vi "Create_Trajectory_Using_TrajectoryLibrary.vi"() -> ()   [LabVIEW 2019]
doc: "This utility creates trajectories based on the robot configuration, constraints and defined waypoints."
uses:
  <vilib>/Rock Robotics/WPI/ThirdParty/JAS_Junk/TrajLib/Trajectory_Library.lvlib
  <vilib>/Rock Robotics/WPI/ThirdParty/JAS_Junk/TrajLib/TypeDef/TRANSLATION2D.ctl
  <vilib>/Rock Robotics/WPI/ThirdParty/JAS_Junk/TrajLib/TypeDef/ROTATION2D.ctl
  <vilib>/Rock Robotics/WPI/ThirdParty/JAS_Junk/TrajLib/TypeDef/POSE2D.ctl
  <vilib>/Rock Robotics/WPI/ThirdParty/JAS_Junk/TrajLib/TypeDef/TRAJ_STATE.ctl
  <vilib>/Rock Robotics/WPI/ThirdParty/JAS_Junk/TrajLib/TypeDef/TRAJECTORY.ctl
  <vilib>/Rock Robotics/WPI/ThirdParty/JAS_Junk/TrajLib/TypeDef/DISPLAY_WEIGHTED_WAYPOINT.ctl
  CreateTrajectoryENUM/TrajCreateUnitsENUM.ctl
  <vilib>/Utility/miscctls.llb/LVCursorListTypeDef.ctl
  <vilib>/Rock Robotics/WPI/ThirdParty/JAS_Junk/TrajLib/TypeDef/TRAJ_CONFIG.ctl
  CreateTrajectoryTypeDef/TrajCreateConfig__V_Internal.ctl
  <vilib>/Utility/xml.llb/Read From XML File(string).vi
  <vilib>/Utility/xml.llb/Write to XML File(string).vi
  <vilib>/Utility/error.llb/DialogType.ctl
  <vilib>/Rock Robotics/WPI/ThirdParty/JAS_Junk/TrajLib/TypeDef/SIMPLE_MOTOR_FF.ctl
  <vilib>/Rock Robotics/WPI/ThirdParty/JAS_Junk/TrajLib/TypeDef/DIFF_DRIVE_KINEMATICS.ctl
panel:
  in  "Update\nConfig":bool
  out "DIFF_DRIVE_KINEMATICS":T1 {"TrackWidth_Meters" format="%20.4f"}
  in  "End Program":bool
  in  "Terminate":bool
  out "FIeldSelectorHasItems":bool
  out "IsCubic":bool
  out "outTRAJECTORY_CONFIG":T2 {"End Velocity" format="%20.4f"; "StartVelocity" format="%20.4f"; "Max Acceleration" format="%20.4f"; "MaxVelocity" format="%20.4f"}
  out "WayPoints_M":T3[](array[typedef]) {"WEIGHT" format="%13.3f"; "ANGLE" format="%13.3f"; "Y" format="%13.3f"; "X" format="%13.3f"}
  out "TRAJECTORY":T4 {"States"."POSE"."ROTATION"."SIN" format="%13.4f"; "States"."POSE"."ROTATION"."COS" format="%13.4f"; "States"."POSE"."ROTATION"."VALUE" format="%13.4f"; "States"."POSE"."TRANSLATION"."Y" format="%14.3f"; "States"."POSE"."TRANSLATION"."X" format="%14.3f"; "TotalTImeSecs" format="%20.3f"}
  in  "Tab Control":T9(tab)
  out "Read Config File Comment":string
  in  "Read Config File Name":path
  in  "ReadConfigFile":bool
  in  "Field Selector":string(combo)
  in  "Units Selector":T10
  in  "MaxVelocity":dbl=50.0 format="%17.1f"
  in  "MaxAcceleration":dbl=40.0 format="%17.1f"
  out "MaxVelocity M/S":dbl=2.0 format="%17.4f"
  out "MaxAcceleration M/S^2":dbl=1.3 format="%17.4f"
  in  "Mech Right Rear":T7={"X"=-0.5, "Y"=0.5} {"Y" format="%14.3f"; "X" format="%14.3f"}
  in  "Mech Left Rear":T7={"X"=-0.5, "Y"=-0.5} {"Y" format="%14.3f"; "X" format="%14.3f"}
  in  "Mech Right Front":T7={"X"=0.5, "Y"=0.5} {"Y" format="%14.3f"; "X" format="%14.3f"}
  in  "Mech Left Front":T7={"X"=0.5, "Y"=-0.5} {"Y" format="%14.3f"; "X" format="%14.3f"}
  in  "Use Centripetal\nAcceleration\nConstaint":bool=TRUE
  in  "Use Diff Drive\nKinematic\nConstraint":bool=TRUE
  in  "Max Voltage":dbl=12.0 format="%20.4f"
  in  "SIMPLE_MOTOR_FF":T11={"Ks"=0.9, "Kv"=0.22199, "Ka"=0.04876, "KnInv"=1.0} {"KnInv" format="%13.4f"; "Ka" format="%13.4f"; "Kv" format="%13.4f"; "Ks" format="%13.4f"}
  in  "Use Diff Drive\nVoltage\nConstraint":bool
  in  "Swerve Wheels":T7[](array[typedef])=[{"X"=0.5, "Y"=-0.5}, {"X"=0.5, "Y"=0.5}, {"X"=-0.5, "Y"=0.5}, {"X"=-0.5, "Y"=-0.5}] {"Y" format="%14.3f"; "X" format="%14.3f"}
  in  "Use Swerve Drive\nKinematics\nConstraint":bool
  in  "Use Mecanum \nDrive\nKinematics\nConstraint":bool
  out "Mech Left Front M":T7 {"Y" format="%14.3f"; "X" format="%14.3f"}
  out "Mech Right Front M":T7 {"Y" format="%14.3f"; "X" format="%14.3f"}
  out "Mech Left Rear M":T7 {"Y" format="%14.3f"; "X" format="%14.3f"}
  out "Mech Right Rear M":T7 {"Y" format="%14.3f"; "X" format="%14.3f"}
  out "SIMPLE_MOTOR_FF M":T11={"Ks"=0.0, "Kv"=0.0, "Ka"=0.0, "KnInv"=1.0} {"KnInv" format="%13.4f"; "Ka" format="%13.4f"; "Kv" format="%13.4f"; "Ks" format="%13.4f"}
  out "Swerve Wheels M":T7[](array[typedef]) {"Y" format="%14.3f"; "X" format="%14.3f"}
  in  "Track Width":dbl=20.866 format="%20.1f"
  out "Track Width M":dbl=0.66 format="%20.4f"
  in  "Max Cent Accel":dbl=20.0 format="%20.1f"
  out "Max Cent Accel M/S^2":dbl=1.0 format="%20.4f"
  in  "Use Rectangular Region\nMax Velocity Constraint":bool
  in  "Rect Reg Top Right":T7 {"Y" format="%14.3f"; "X" format="%14.3f"}
  in  "REct Reg Bot Left":T7 {"Y" format="%14.3f"; "X" format="%14.3f"}
  in  "Region Max Speed (Units/Sec)":dbl=40.0 format="%20.4f"
  out "Rect Reg Top Right M":T7 {"Y" format="%14.3f"; "X" format="%14.3f"}
  out "Rect Reg Bot Left M":T7 {"Y" format="%14.3f"; "X" format="%14.3f"}
  out "Region Max Speed M/Sec":dbl
  in  "Remove Current\nWaypoint":bool
  in  "Add New\nWaypoint":bool
  in  "WayPoints":T3[](array[typedef])=[{"X"=15.0, "Y"=105.0, "ANGLE"=-45.0, "WEIGHT"=12.0}, {"X"=105.0, "Y"=65.0, "ANGLE"=0.0, "WEIGHT"=12.0}, {"X"=210.0, "Y"=106.0, "ANGLE"=45.0, "WEIGHT"=12.0}, {"X"=350.0, "Y"=105.0, "ANGLE"=-45.0, "WEIGHT"=12.0}] {"WEIGHT" format="%13.3f"; "ANGLE" format="%13.3f"; "Y" format="%13.3f"; "X" format="%13.3f"}
  in  "Spline Type":enum32{"Radio Selection 1", "Radio Selection 2"}(radio)
  in  "Reverse":bool
  in  "UseWeights":bool
  in  "Calculate\nTrajectory":bool
  out "Trajectory\nCompleted\nError Free":bool
  out "Trajectory calculation error":errorcluster
  out "Position":cluster{dbl[], dbl[]}[](graph)
  out "Index":i32
  out "2D Picture":picture
  out "Trajectory Data":cluster{dbl[], dbl[]}[](graph)
  out "differential \ndrive \nmax speed":dbl format="%15.1f"
  out "Traj States\nSize":i32
  out "Trajectory States":T5[](array[typedef]) {"POSE"."ROTATION"."SIN" format="%13.4f"; "POSE"."ROTATION"."COS" format="%13.4f"; "POSE"."ROTATION"."VALUE" format="%13.4f"; "POSE"."TRANSLATION"."Y" format="%14.3f"; "POSE"."TRANSLATION"."X" format="%14.3f"}
  in  "Trajectory JSON File Name":path
  in  "PathWeaver Length Units":T12(radio)
  in  "WriteJSONFile":bool
  in  "Trajectory Type":enum32{"Radio Selection 1", "Radio Selection 2"}(radio)
  in  "Trajectory File Comment":string
  in  "Trajectory CSV File Name":path
  in  "WriteTrajFile":bool
  in  "Write Config File Comment":string
  in  "Write Config File Name":path
  in  "WriteConfigFile":bool
  # "Create Trajectory  (Use LabVIEW trajectory library)"
  # "Instructions:  \n----------------\n\nThis utility will create a trajectory, show the data on the various tabs, and optionally write a \"field absolute\" or \"robot relative\" trajectory to a file. \nTo use this utility:\n\n    1) Read all of these instructions!\n    2) Define the robot's physical data on the \"Robot Data\" tab.  \n    3) Define the robot's movement constraints on the \"Constraints\" and \"Constraints 2\" tab.  \n    4) Define the trajectory on the \"Define/Create Trajectory\" tab.  These are the beginning and ending positions/headings, and internal positions/headings.  \n         Cubic splines only use the first and last \"angle\".  The other internal \"angles\" are calculated.  Quintic splines use all the defined angles.\n    5) Press the \"Calculate Trajectory\".  If a good trajectory was calculated it will be displayed.  If no errors are generated the Trajectory Complete\n         light will be on.  Errors will be displayed in the error indicator.  The path can be recalculated many times before performing any other action.\n\nAfter a Trajectory has been calculated, the \"trajectory can be written to a file.  The absolute path is converted to a robot relative trajectory.  To do this:\n    1) Enter a comment to be included in the file.  Anything can be entered.\n    2) Select the file name.\n    3) Press \"Create CSV Trajectory File\"  If an error occurs it will be displayed in the File Creation Error indicator.\n\nTo:\n  --  Move a WayPoint  -- Left click the waypoint and drag it using the mouse.\n  --  Rotate a WayPoint  -- Left click the waypoint to select, then use the mouse wheel to increase or decrease the heading\n  --  Change WayPoint weight  -- Left click the waypoint to select, then use CTRL key and mouse wheel to increase or decrease the weight.\n\nNotes:\n--------\n- All the robot parameters, path, and field dimensions are in UNITS, and DEGREES.  Select UNITS from the \"Robot Data\" page.  The resulting  \n  trajectory is converted to METERS, and RADIANS to match the rest of this library!\n- 2019 playing field size - width: 26 ft 11.25 In = 323.25 in , length: 52 ft 5.25 in = 629.25 in  (This changes from year to year.  Larger fields are allowed.)\n\nAcknowlegements\n------------------------\n- Nathanael Cornell from FRC team 5205 added the initial code to visually move and rotate waypoints."
  # "Read Trajectory Waypoints and Configuration from File"
  # "ROBOT DATA"
  # "UNITS/SEC"
  # "Meters/SEC"
  # "UNITS/SEC^2"
  # "Meters/SEC^2"
  # "Simulated diff drive robot max speed is: 68.266 Inches/Second"
  # "UTILITY CONFIGURATION"
  # "Diff Kinematics Constraint"
  # "Centripetal Accel Constraint"
  # "Diff Voltage Constraint"
  # "UNITS"
  # "UNITS/SEC^2"
  # "VOLTS"
  # "METERS"
  # "METERS/SEC^2"
  # "Distance is:\nUNITS"
  # "Simulated robot wheelbase is 20.87 in"
  # "Ks = Volts\nKv = VoltSec/Meter\nKa = Volt(Sec^2)/Meter"
  # "Swerve Kinematics Constraint"
  # "Mechanum Kinematics Constraint"
  # "Values\nare \nUNITS"
  # "Values\nare \nUNITS"
  # "Rectangular Region Constraint  - Max Velocity Constraint"
  # "Values\nare \nUNITS"
  # "TRAJECTORY DEFINITION"
  # "To delete array elements or the entire array, right click on the array or element, select Data Operations, then select the action to be performed."
  # "UNITS, UNITS, DEGREES, SCALAR"
  # "INCHES/SEC"
  # "Write Trajectory to File   -   CSV, and / or JSON"
  # "Write Trajectory Waypoints and Configuration to File"
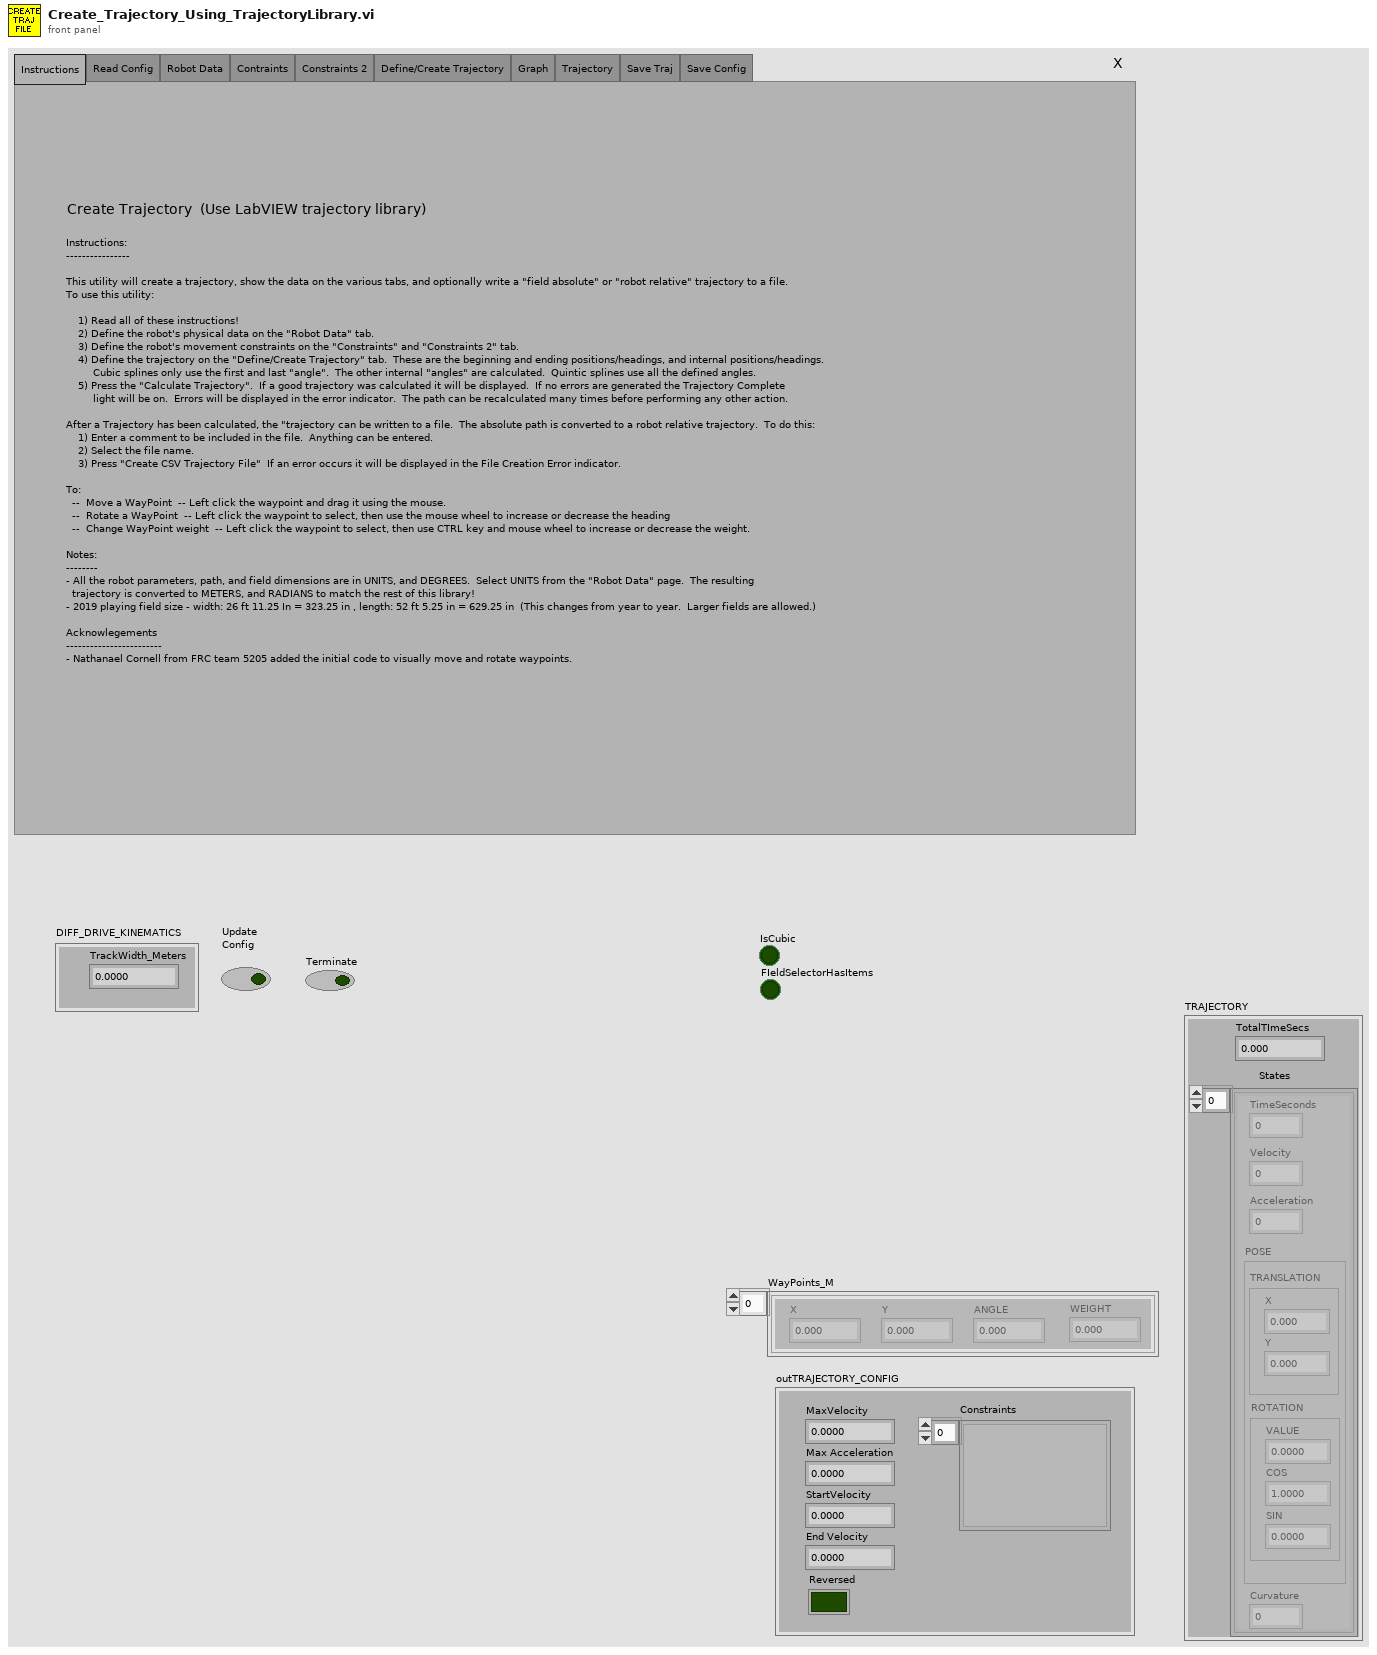
[diagram p1: front panel]
types:
  T1 = typedef "Trajectory_Library.lvlib/DIFF_DRIVE_KINEMATICS.ctl" = cluster{"TrackWidth_Meters":dbl}
  T2 = typedef "Trajectory_Library.lvlib/TRAJ_CONFIG.ctl" = cluster{"MaxVelocity":dbl, "Max Acceleration":dbl, "StartVelocity":dbl, "End Velocity":dbl, "Reversed":bool, "Constraints":variant[]}
  T3 = typedef "Trajectory_Library.lvlib/DISPLAY_WEIGHTED_WAYPOINT.ctl" = cluster{"X":dbl, "Y":dbl, "ANGLE":dbl, "WEIGHT":dbl}
  T4 = typedef "Trajectory_Library.lvlib/TRAJECTORY.ctl" = cluster{"TotalTImeSecs":dbl, "States":T5[]}
  T5 = typedef "Trajectory_Library.lvlib/TRAJ_STATE.ctl" = cluster{"TimeSeconds":dbl, "Velocity":dbl, "Acceleration":dbl, "POSE":T6, "Curvature":dbl}
  T6 = typedef "Trajectory_Library.lvlib/POSE2D.ctl" = cluster{"TRANSLATION":T7, "ROTATION":T8}
  T7 = typedef "Trajectory_Library.lvlib/TRANSLATION2D.ctl" = cluster{"X":dbl, "Y":dbl}
  T8 = typedef "Trajectory_Library.lvlib/ROTATION2D.ctl" = cluster{"VALUE":dbl, "COS":dbl, "SIN":dbl}
  T9 = enum32{"Instructions", "Read Config", "Robot Data", "Contraints", "Constraints 2", "Define/Create Trajectory", "Graph", "Trajectory", "Save Traj", "Save Config"}
  T10 = typedef "TrajCreateUnitsENUM.ctl" = enum16{"Inches", "Feet", "Centimeters", "Meters"}
  T11 = typedef "Trajectory_Library.lvlib/SIMPLE_MOTOR_FF.ctl" = cluster{"Ks":dbl, "Kv":dbl, "Ka":dbl, "KnInv":dbl}
  T12 = enum32{"Radio Selection 1", "Radio Selection 2", "Radio Selection 3", "Radio Selection 4", "Radio Selection 5"}
  T13 = typedef "LVCursorListTypeDef.ctl" = cluster{"Name":string, "Color":u32, "Style":u8, "Point Style":u8, "Name Visible":bool, "Allow Drag":bool, "Cursor Mode":u32, "Plot":i32, "Index":i32, "Position":cluster{"X":dbl, "Y":dbl}, "X Scale":u32, "Y Scale":u32, "Watch Plots":i32[], "Watch All Plots":bool, "Plot Area":i32, "Label Offset":cluster{"X":dbl, "Y":dbl}}[]
  T14 = enum8{"Enabled", "Disabled", "Disabled and Grayed Out"}
  T15 = cluster{"Name":string, "Color":u32, "Style":u8, "Point Style":u8, "Name Visible":bool, "Allow Drag":bool, "Cursor Mode":u32, "Plot":i32, "Index":i32, "Position":cluster{"X":dbl, "Y":dbl}, "X Scale":u32, "Y Scale":u32, "Watch Plots":i32[], "Watch All Plots":bool, "Plot Area":i32, "Label Offset":cluster{"X":dbl, "Y":dbl}}
  T16 = typedef "TrajCreateConfig__V_Internal.ctl" = cluster{"Write Config File Name":path, "Write Config File Comment":string, "WayPoints":T3[], "TRAJECTORY_CONFIG":T2, "IsCubic":bool, "Units Selector":T10, "UseWeights":bool, "FieldName":string}
  T17 = typedef "Trajectory_Library.lvlib/SWERVE_DRIVE_KINEMATICS.ctl" = cluster{"NumModules":i32, "InverseKinematics":T18, "ForwardKinematics":T18, "Modules":T7[], "PrevCoR":T7, "SavedModuleStates":T19[]}
  T18 = typedef "NI_Matrix.lvlib/RealMatrix.ctl" = dbl[][]
  T19 = typedef "Trajectory_Library.lvlib/SWERVE_DRIVE_MODULE_STATE.ctl" = cluster{"Speed":dbl, "Angle":T8}
  T20 = typedef "Trajectory_Library.lvlib/MECA_DRIVE_KINEMATICS.ctl" = cluster{"FrontLeft":T7, "FrontRight":T7, "RearLeft":T7, "RearRight":T7, "InverseKinematics":T18, "ForwardKinematics":T18, "PrevCoR":T7}
  T21 = typedef "Trajectory_Library.lvlib/TRAJ_CONSTRAINT_MAX_VELOCITY.ctl" = cluster{"Max Velocity":dbl, "IM UNIQUE":bool}
  T22 = typedef "Trajectory_Library.lvlib/TRAJ_CONSTRAINT_RECT_REGION.ctl" = cluster{"BottomLeftPoint":T7, "TopRightPoint":T7, "Constraint":variant, "Constraint Type":T23}
  T23 = typedef "Trajectory_Library.lvlib/TRAJ_CONSTRAINT_TYPES_ENUM.ctl" = enum16{"UNDEFINED", "DIFF DRIVE KINEMATICS", "DIFF DRIVE VOLTAGE", "CENTRIPITAL ACCEL", "MECA DRIVE KINEMATICS", "SWERVE DRIVE KINEMATICS", "MAXIMUM VELOCITY", "ELLIPTICAL REGION", "RECTANGULAR REGION"}
  T24 = typedef "DialogType.ctl" = u16
  T25 = typedef "Trajectory_Library.lvlib/TRAJ_CONSTRAINT_DIIF_DRIVE_KINEMATICS.ctl" = cluster{"Max Speed (M/S)":dbl, "DIFF_DRIVE_KINEMATICS":T1, "Max Accel (M/S2)":dbl}
  T26 = typedef "Trajectory_Library.lvlib/TRAJ_CONSTRAINT_CENTRIPETAL_ACCEL.ctl" = cluster{"Max Cent Accel":dbl}
  T27 = typedef "Trajectory_Library.lvlib/TRAJ_CONSTRAINT_DIIF_DRIVE_VOLTAGE.ctl" = cluster{"Max Voltage":dbl, "DIFF_DRIVE_KINEMATICS":T1, "SIMPLE_MOTOR_FF":T11}
  T28 = typedef "Trajectory_Library.lvlib/TRAJ_CONSTRAINT_MECA_DRIVE_KINEMATICS.ctl" = cluster{"Max Speed (M/S)":dbl, "MECA_DRIVE_KINEMATICS":T20}
  T29 = typedef "Trajectory_Library.lvlib/TRAJ_CONSTRAINT_SWERVE_DRIVE_KINEMATICS.ctl" = cluster{"Max Speed (M/S)":dbl, "SwerveKinematics":T17}
  T30 = typedef "TrajCreateConfig_V5.ctl" = cluster{"Write Config File Name":path, "Write Config File Comment":string, "WayPoints":T3[], "TRAJECTORY_CONFIG_V4":T31, "IsCubic":bool, "Units Selector":T10, "UseWeights":bool, "FieldName":string, "Rect Region Exists":bool, "RectRegionBotLeft":T7, "RectRegionTopRight":T7, "Rect Region Max Speed":dbl}
  T31 = typedef "TrajCreateTrajConfig_V4.ctl" = cluster{"MaxVelocity":dbl, "Max Acceleration":dbl, "StartVelocity":dbl, "End Velocity":dbl, "Reversed":bool, "DiffDrKineConstntDefined":bool, "CentAcellConstntDefined":bool, "DiffDrVoltConstntDefined":bool, "DIFF_DRIVE_KINE_CONSTRAINT":T25, "CENTRIPETAL_ACCEL_CONSTRAINT":T26, "SwerveDrKineConstntDefined":bool, "SWERVE_DRIVE_KINE_CONSTRAINT":T29, "DIFF_DRIVE_VOLTAGE_CONSTRAINT":T27, "MECANUM_DRIVE_KINE_CONSTRAINT":T28, "MecanumDrKineConstntDefined":bool}
  T32 = cluster{"Shift":bool, "Ctrl":bool, "Alt":bool, "Cmd":bool, "Opt":bool}
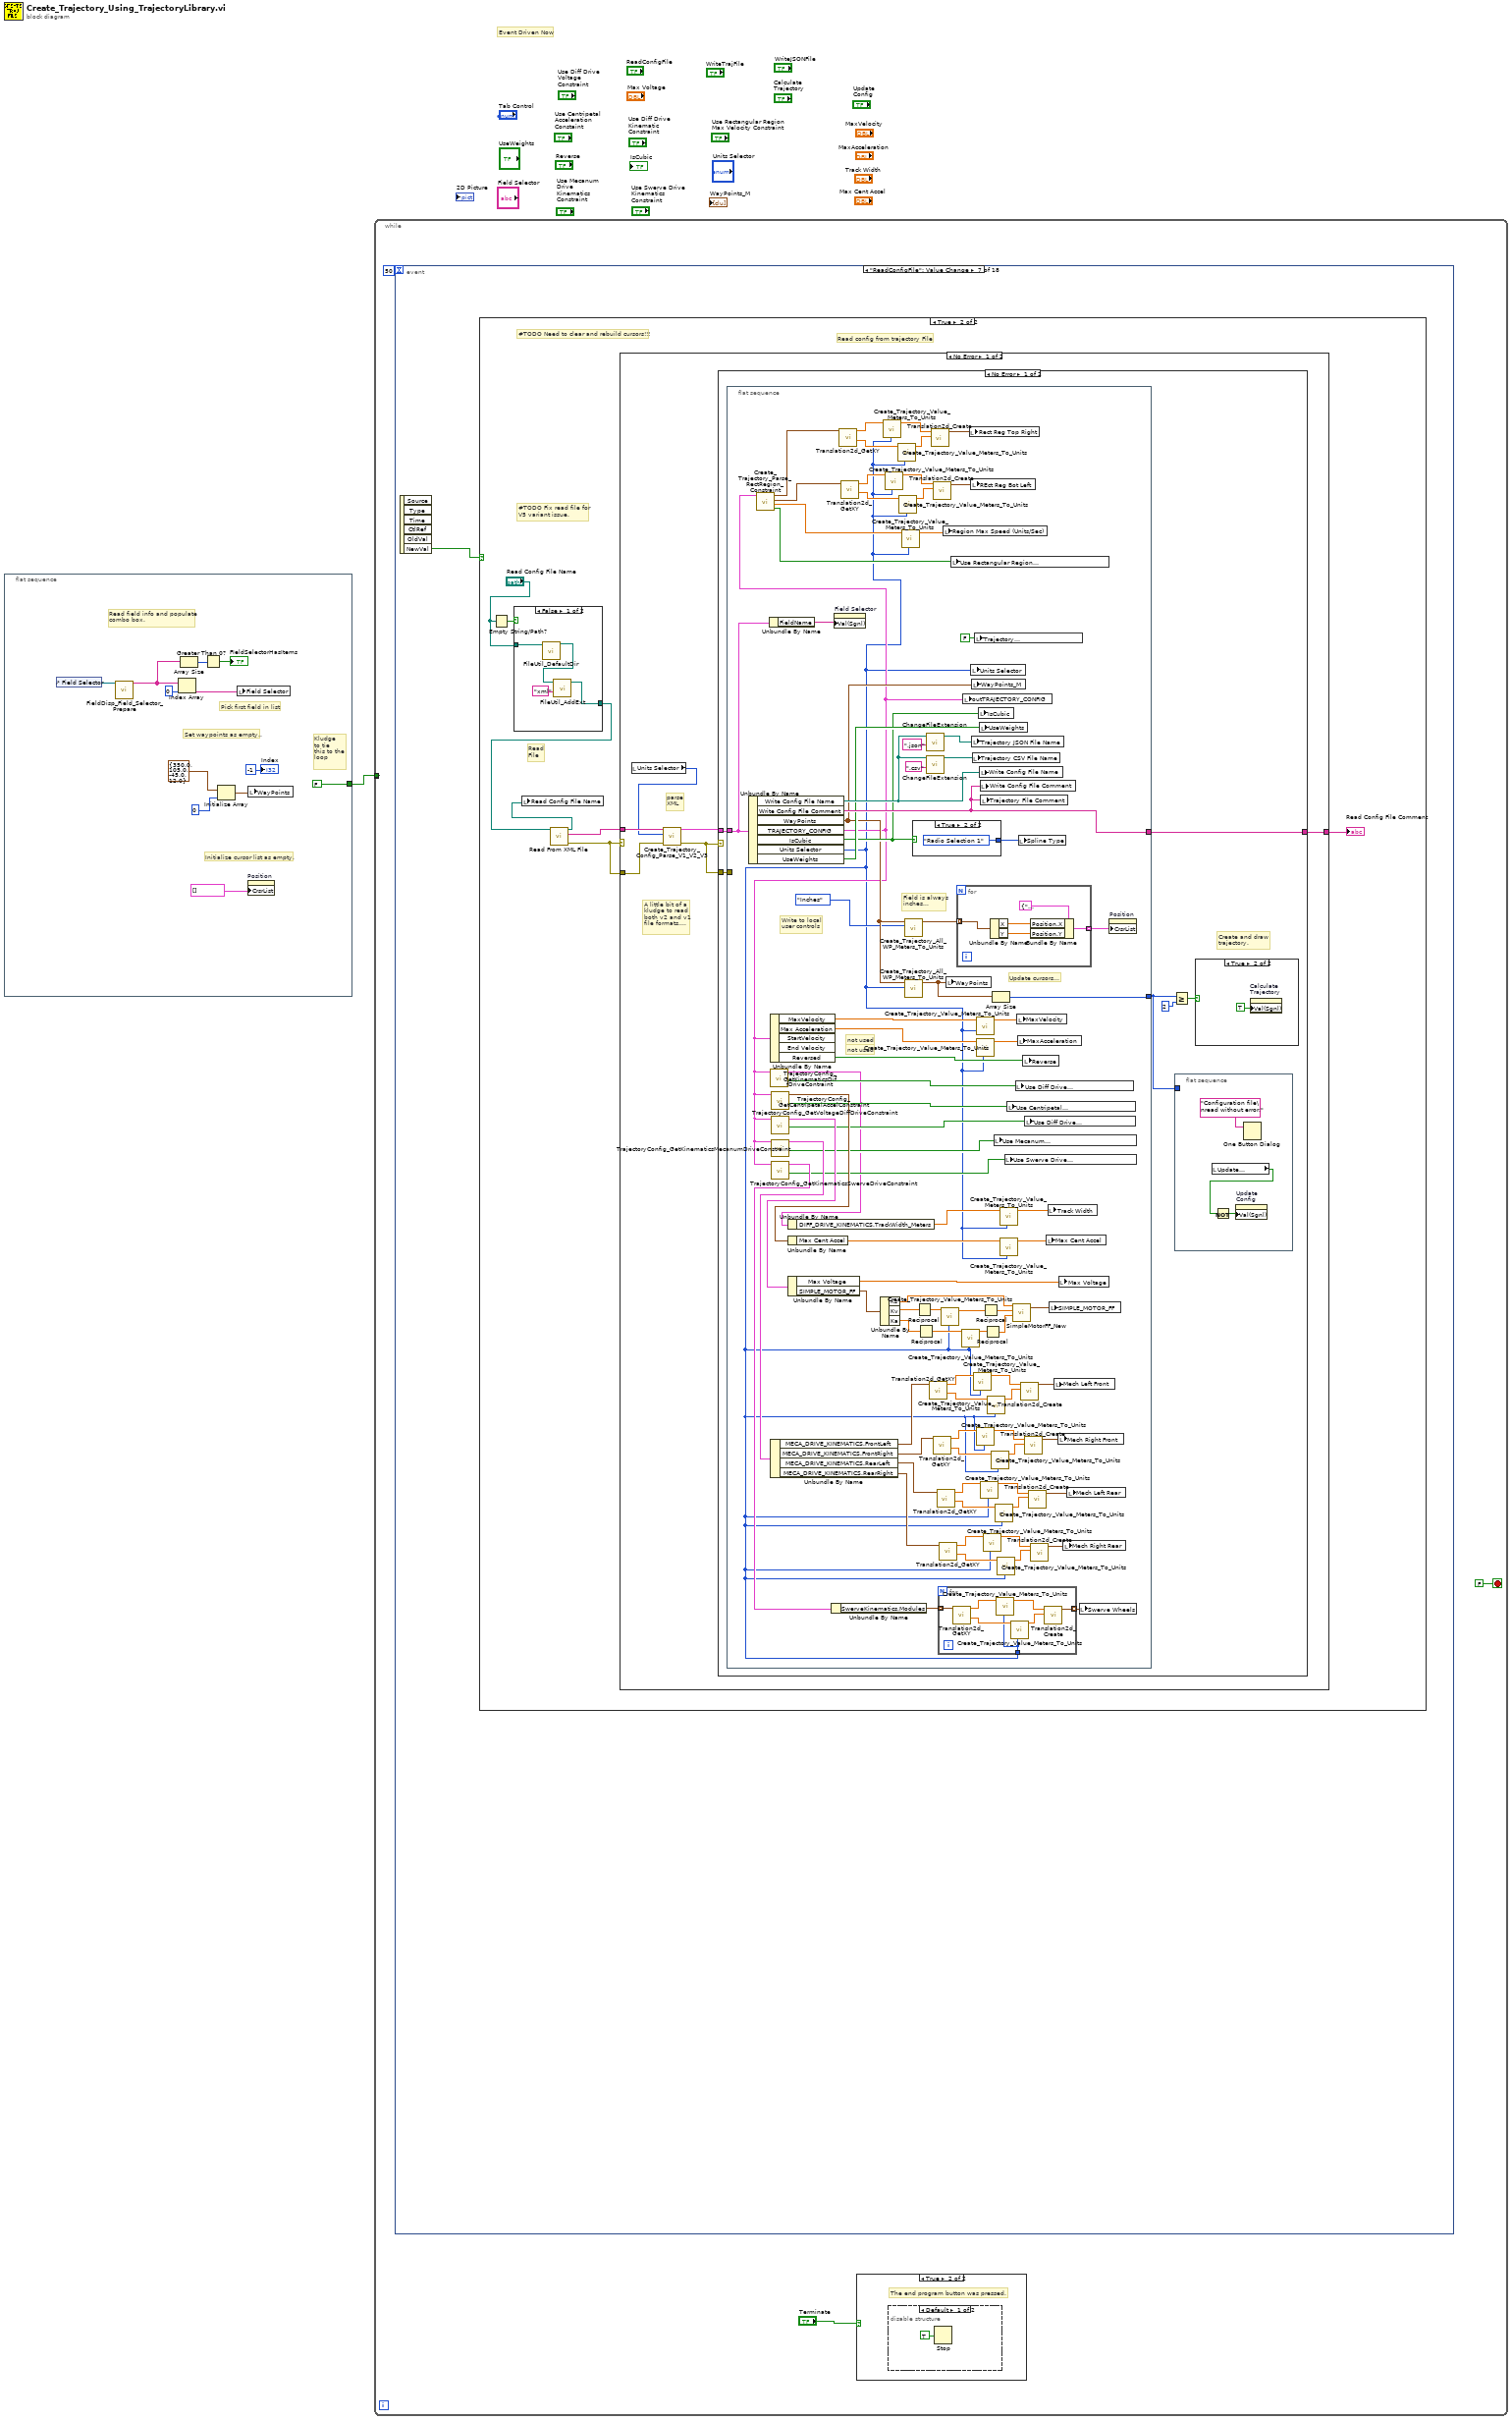
[diagram p0: block diagram]
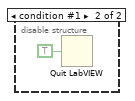
[diagram p3: hidden frame]
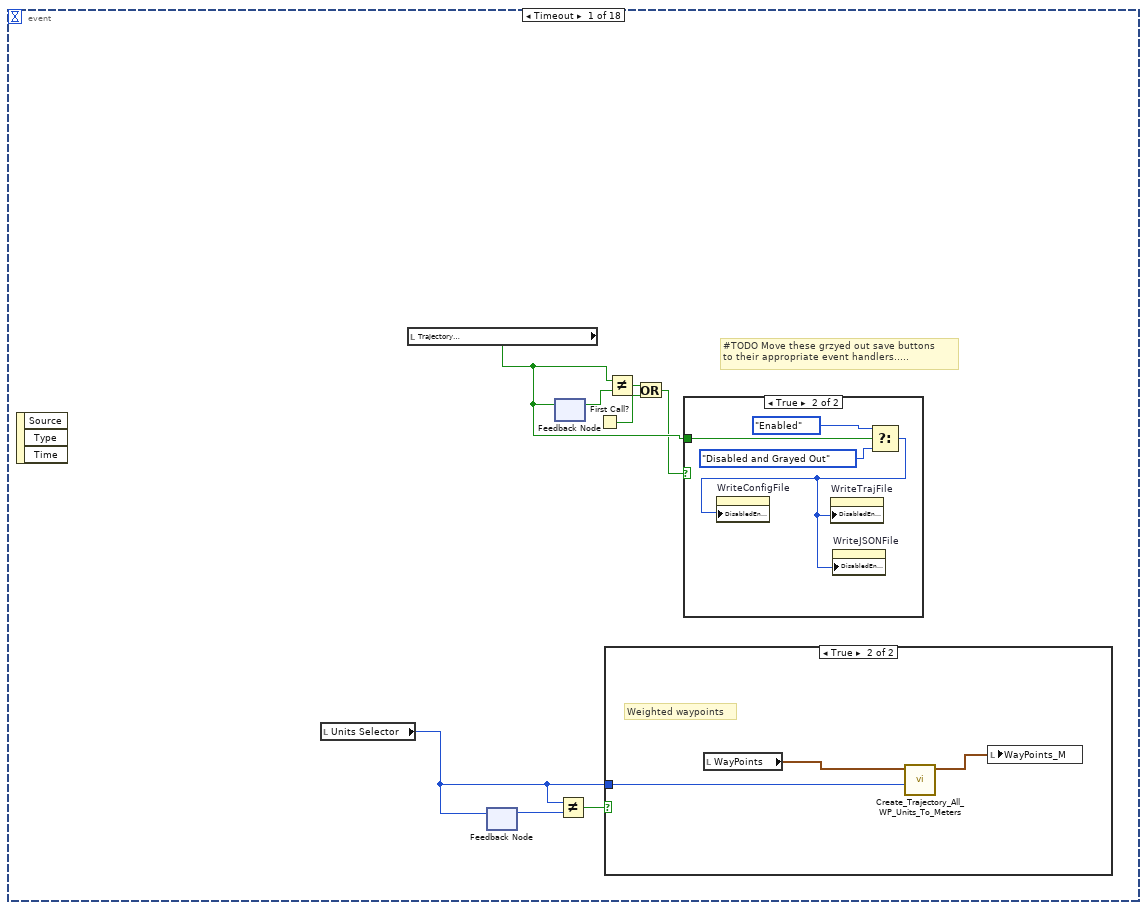
[diagram p4: hidden frame]
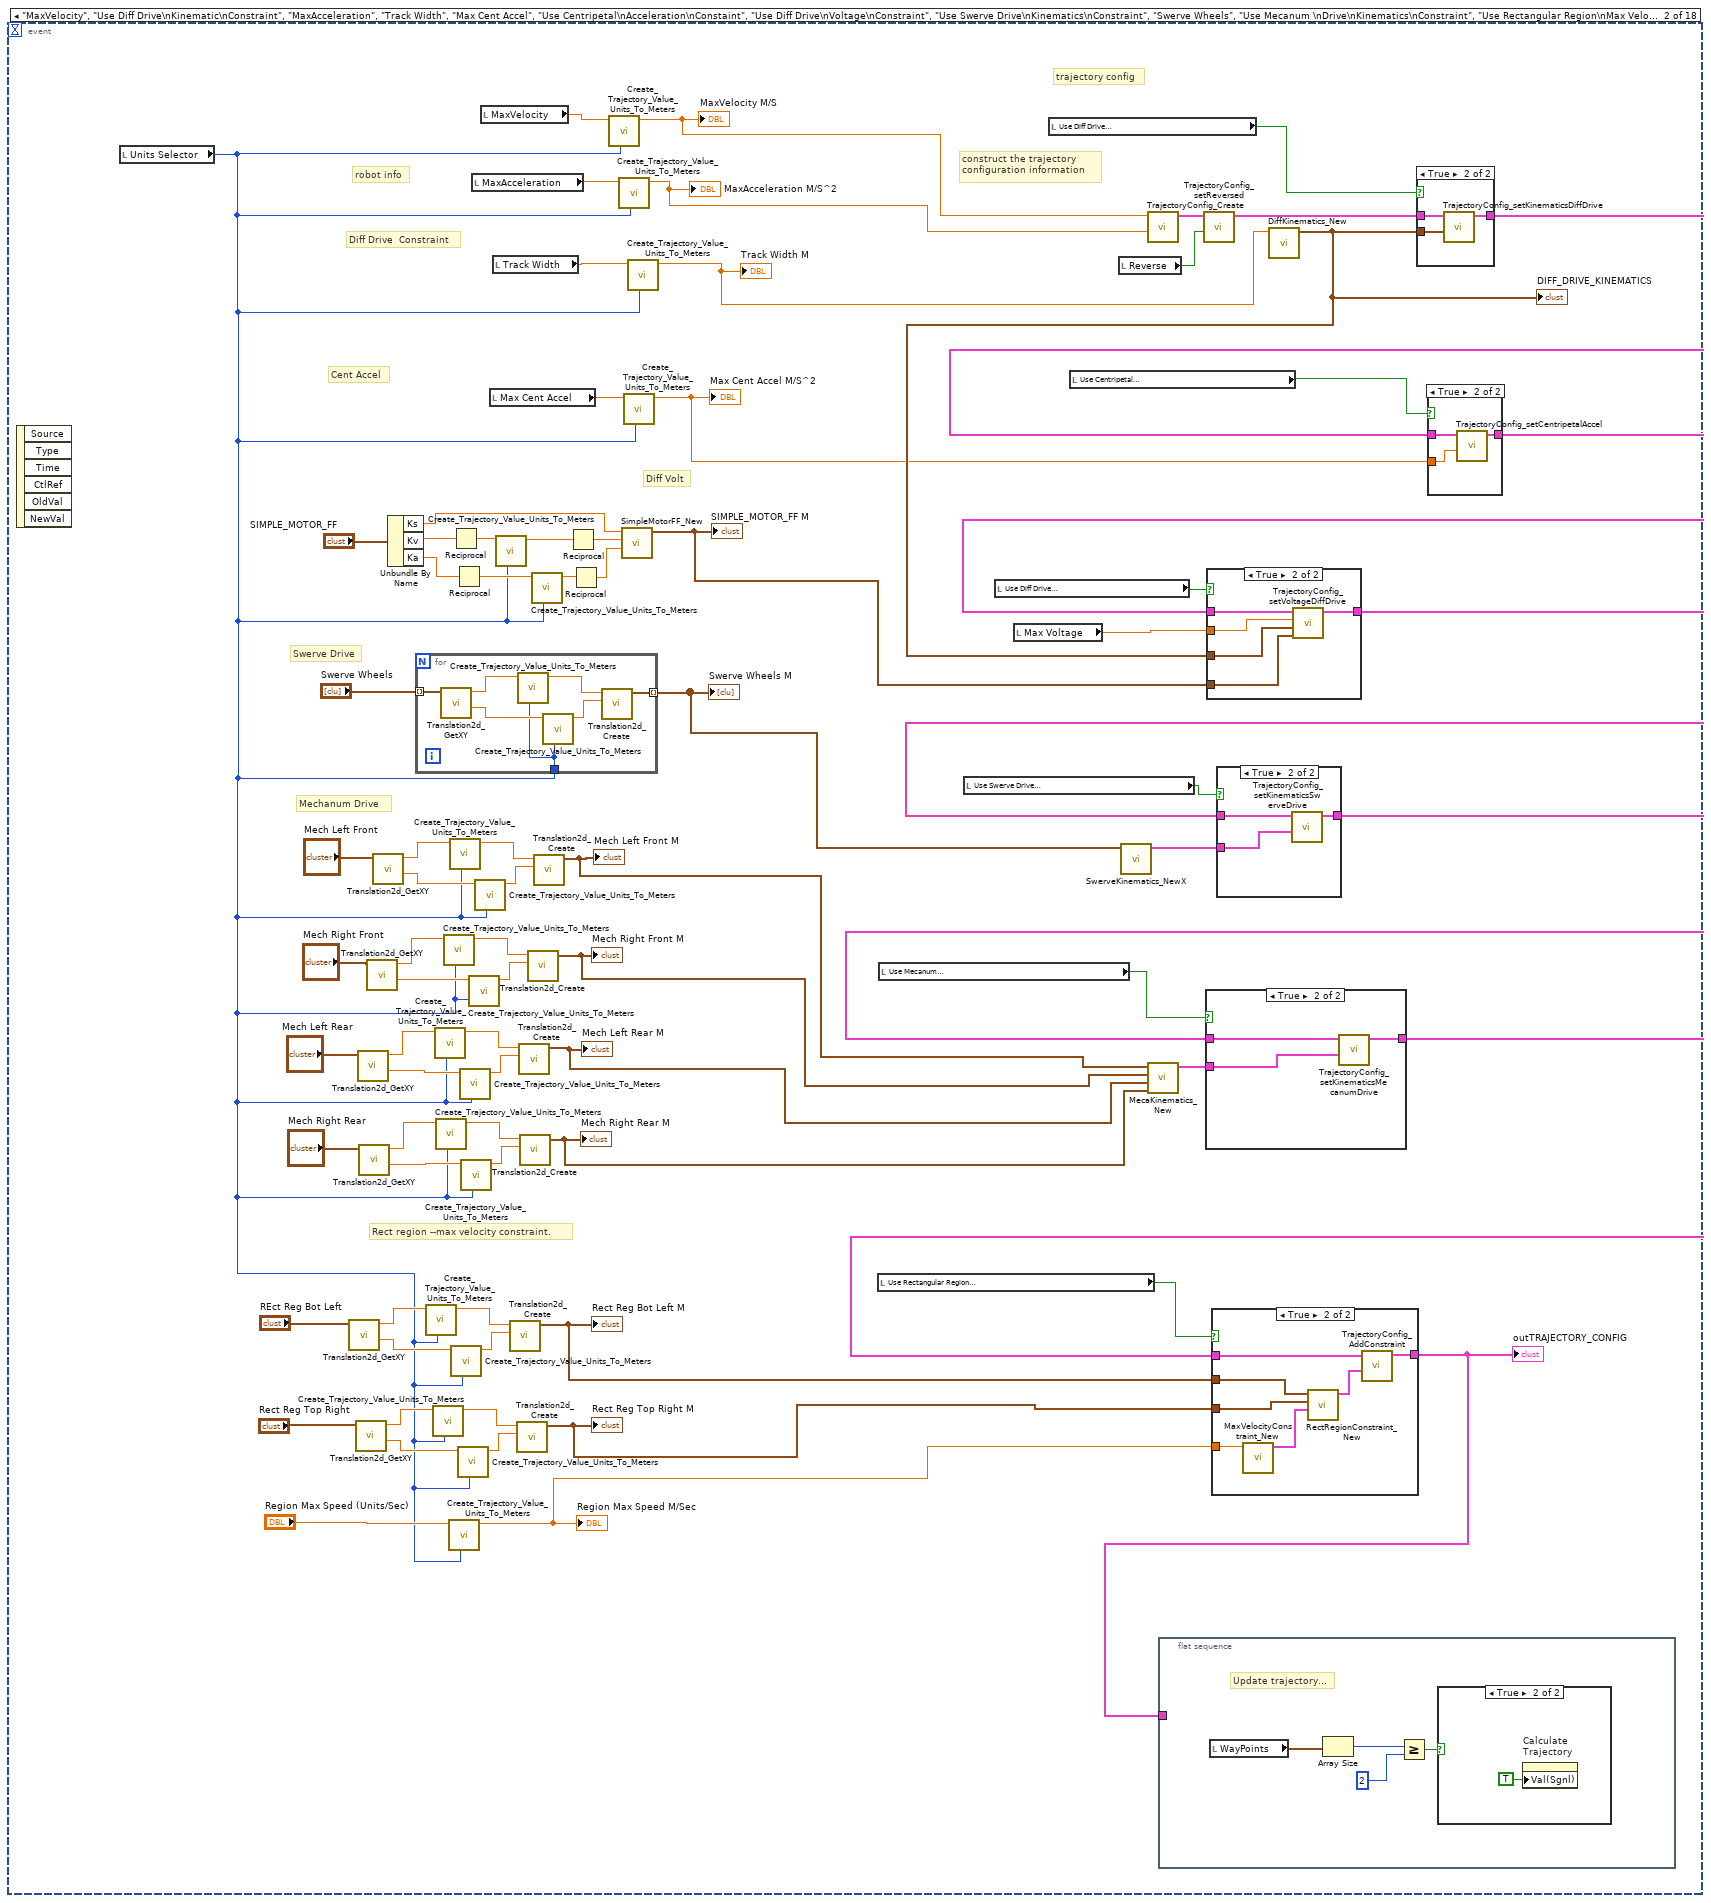
[diagram p7: hidden frame]
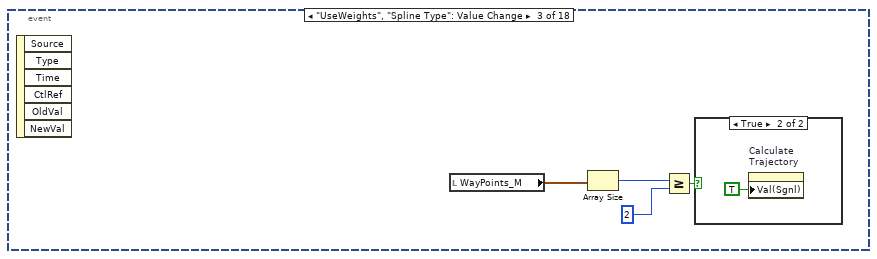
[diagram p15: hidden frame]
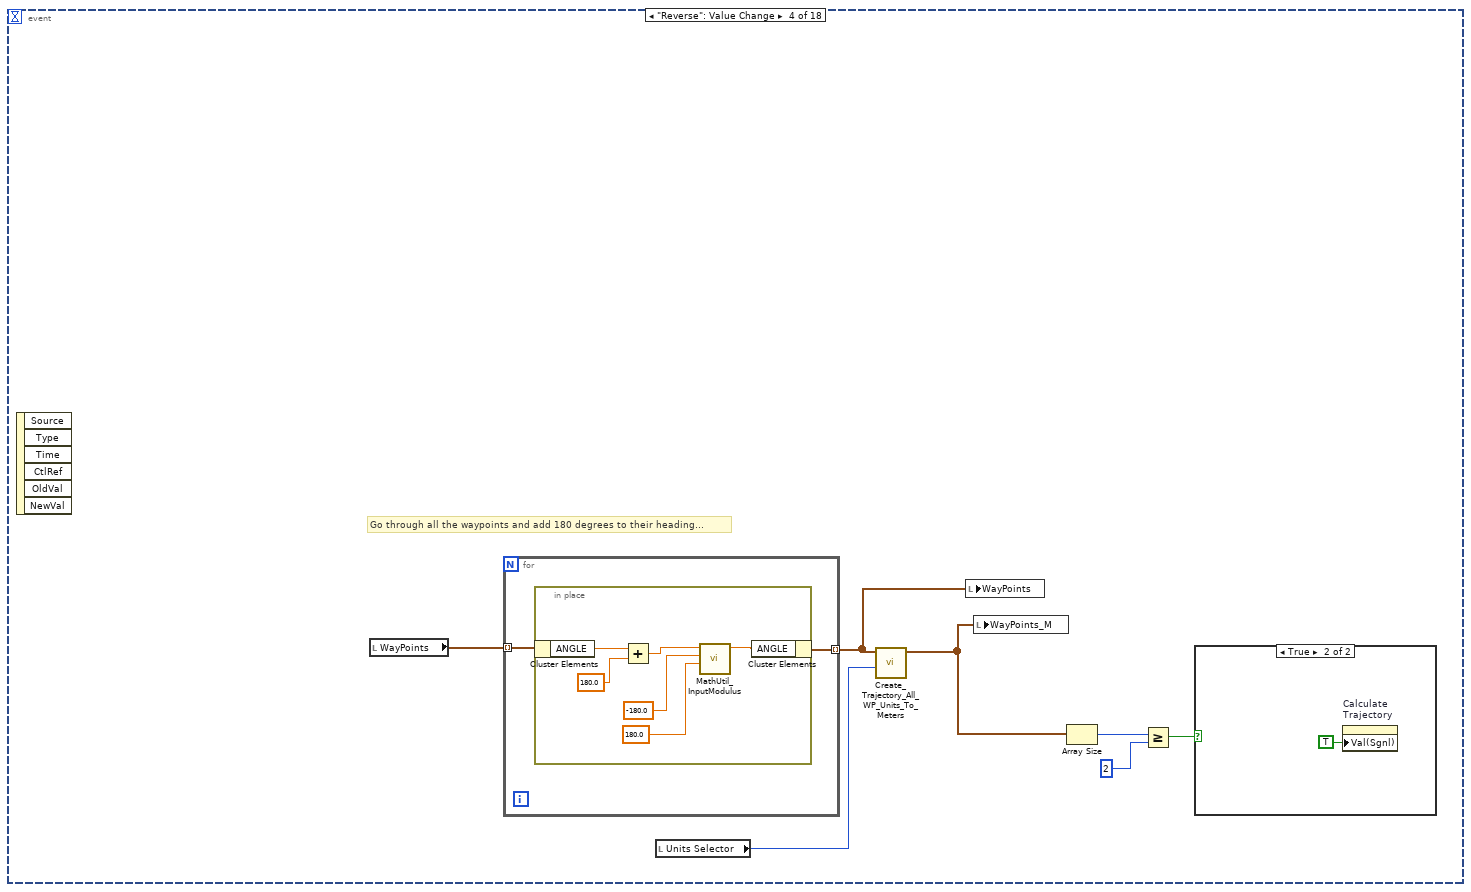
[diagram p17: hidden frame]
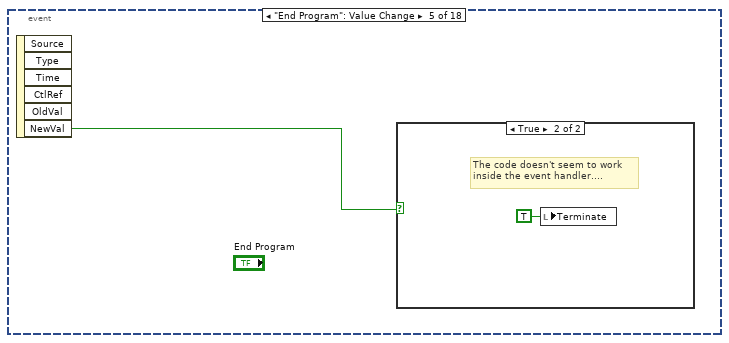
[diagram p19: hidden frame]
diagram:
  # "Event Driven Now"
  n1 = flat-sequence {
    tunnel: [FALSE] -> w1
    frame #0 {
      # "Pick first field in list"
      # "Read field info and populate\ncombo box."
      # "Kludge\nto tie\nthis to the\nloop"
      # "Initialize cursor list as empty."
      # "Set waypoints as empty.."
      n2 = control-ref of="Field Selector"() -> (w6:refnum<vi>)
      n3 = call <vilib>:"FieldDisp_Field_Selector_Prepare.vi"("ComboBox Ref"=w6) -> ("section names"=w7:string[])  [unwired: 9 in, 1 out]
      n4 = Index Array(array=w7, index=0) -> (element=w5:string)
      n5 = Array Size(array=w7) -> (size(s)=w3:i32)
      n6 = Greater Than 0?(x=w3) -> (x > 0?=→"FIeldSelectorHasItems":bool)
      n7 = Initialize Array(T3 {"X"=350.0, "Y"=105.0, "ANGLE"=-45.0, "WEIGHT"=12.0} ("path"), 0 ("dimension size")) -> (w11:T3[])
      n8 = local write "Field Selector"(w5) -> ()
      n9 = property on="Position" class="XYGraph (strict)"("CrsrList"=T13 [] ("Cursor List")) -> ()  [unwired: 2 in, 2 out]
      n10 = local write "WayPoints"(w11) -> ()
      "Index" <- -1 ("Index")
    }
  }
  n11 = while {
    tunnel: [w15] -> _
    tunnel: w1 -> [w15]
    stop <- FALSE stop-if-true
    n12 = event shown="[6] \"ReadConfigFile\": Value Change" {
      selector: _ -> [_ _ _ _ _ _ _ _ _ _ _ _ _ _ _ _ _ _]
      dyn-events: _ -> [_ _ _ _ _ _ _ _ _ _ _ _ _ _ _ _ _ _]
      timeout: 50 -> [_ _ _ _ _ _ _ _ _ _ _ _ _ _ _ _ _ _]
      event Timeout {
        # "#TODO Move these grzyed out save buttons\nto their appropriate event handlers....."
        n13 = event-data() -> ()  [unwired: 1 in, 3 out]
        n14 = local read "Units Selector"() -> (w20:T10)
        n15 = local read "Trajectory\nCompleted\nError Free"() -> (w27:bool)
        n16 = feedback-in #1(w20) -> ()
        n17 = feedback #1() -> (w21:T10)  [unwired: 1 in]
        n18 = feedback #2() -> (w23:bool)  [unwired: 1 in]
        n19 = feedback-in #2(w27) -> ()
        n20 = Not Equal?(x=w20, y=w21) -> (x != y?=w22:bool)
        n21 = First Call?() -> (First Call?: T/F=w25:bool)
        n22 = case shown="True" w22 {
          tunnel: w20 -> [_ w30]
          frame False {
          }
          frame True {
            # "Weighted waypoints"
            n23 = local read "WayPoints"() -> (w28:T3[])
            n24 = call "Create_Trajectory_All_WP_Units_To_Meters.vi"("Units Selector"=w30, "WayPoints"=w28) -> ("Array"=w29:T3[])  [unwired: 9 in]
            n25 = local write "WayPoints_M"(w29) -> ()
          }
        }
        n26 = Not Equal?(x=w27, y=w23) -> (x != y?=w24:bool)
        n27 = Or(x=w24, y=w25) -> (x .or. y?=w26:bool)
        n28 = case shown="True" w26 {
          tunnel: w27 -> [_ w34]
          frame False {
          }
          frame True {
            n29 = Select(t=T14."Enabled" ("Disabled"), s=w34, f=T14."Disabled and Grayed Out" ("Disabled")) -> (s? t:f=w31:T14)
            n30 = property on="WriteConfigFile" class="Bool"("DisabledEnum"=w31) -> ()  [unwired: 2 in, 2 out]
            n31 = property on="WriteTrajFile" class="Bool (strict)"("DisabledEnum"=w31) -> ()  [unwired: 2 in, 2 out]
            n32 = property on="WriteJSONFile" class="Bool (strict)"("DisabledEnum"=w31) -> ()  [unwired: 2 in, 2 out]
          }
        }
      }
      event "MaxVelocity", "Use Diff Drive\nKinematic\nConstraint", "MaxAcceleration", "Track Width", "Max Cent Accel", "Use Centripetal\nAcceleration\nConstaint", "Use Diff Drive\nVoltage\nConstraint", "Use Swerve Drive\nKinematics\nConstraint", "Swerve Wheels", "Use Mecanum \nDrive\nKinematics\nConstraint", "Use Rectangular Region\nMax Velocity Constraint", "Region Max Speed (Units/Sec)", "Max Voltage", "Update\nConfig": Value Change {
        # "construct the trajectory\nconfiguration information"
        # "Rect region --max velocity constraint."
        # "Swerve Drive"
        # "Mechanum Drive"
        # "Diff Volt"
        # "Cent Accel"
        # "robot info"
        # "Diff Drive  Constraint"
        # "trajectory config"
        n33 = event-data() -> ()  [unwired: 1 in, 6 out]
        n34 = local read "Units Selector"() -> (w67:T10)
        n35 = call <vilib>:"Translation2d_GetXY.vi"("In Translation"="REct Reg Bot Left") -> ("Y"=w77:dbl, "X"=w75:dbl)  [unwired: 9 in]
        n36 = call <vilib>:"Translation2d_GetXY.vi"("In Translation"="Rect Reg Top Right") -> ("Y"=w73:dbl, "X"=w71:dbl)  [unwired: 9 in]
        n37 = call <vilib>:"Translation2d_GetXY.vi"("In Translation"="Mech Left Rear") -> ("Y"=w91:dbl, "X"=w89:dbl)  [unwired: 9 in]
        n38 = call <vilib>:"Translation2d_GetXY.vi"("In Translation"="Mech Right Rear") -> ("Y"=w96:dbl, "X"=w94:dbl)  [unwired: 9 in]
        n39 = call <vilib>:"Translation2d_GetXY.vi"("In Translation"="Mech Right Front") -> ("Y"=w86:dbl, "X"=w84:dbl)  [unwired: 9 in]
        n40 = call <vilib>:"Translation2d_GetXY.vi"("In Translation"="Mech Left Front") -> ("Y"=w81:dbl, "X"=w79:dbl)  [unwired: 9 in]
        n41 = Unbundle By Name("SIMPLE_MOTOR_FF") -> ("Ks"=w101:dbl, "Kv"=w102:dbl, "Ka"=w109:dbl)
        n42 = for {
          tunnel: "Swerve Wheels" -> [w151] mode=indexing
          tunnel: [w150] -> w48 mode=indexing
          tunnel: w67 -> [w149]
          n43 = call <vilib>:"Translation2d_GetXY.vi"("In Translation"=w151) -> ("Y"=w153:dbl, "X"=w155:dbl)  [unwired: 9 in]
          n44 = call "Create_Trajectory_Value_Units_To_Meters.vi"("Units Selector"=w149, "Units"=w155) -> ("Meters"=w154:dbl)  [unwired: 9 in]
          n45 = call "Create_Trajectory_Value_Units_To_Meters.vi"("Units Selector"=w149, "Units"=w153) -> ("Meters"=w152:dbl)  [unwired: 9 in]
          n46 = call <vilib>:"Translation2d_Create.vi"("Y"=w152, "X"=w154) -> ("TRANSLATION"=w150:T7)  [unwired: 9 in]
        }
        "Swerve Wheels M" <- w48
        n47 = call "Create_Trajectory_Value_Units_To_Meters.vi"("Units Selector"=w67, "Units"=w75) -> ("Meters"=w76:dbl)  [unwired: 9 in]
        n48 = call "Create_Trajectory_Value_Units_To_Meters.vi"("Units Selector"=w67, "Units"=w71) -> ("Meters"=w72:dbl)  [unwired: 9 in]
        n49 = call "Create_Trajectory_Value_Units_To_Meters.vi"("Units Selector"=w67, "Units"=w89) -> ("Meters"=w90:dbl)  [unwired: 9 in]
        n50 = call "Create_Trajectory_Value_Units_To_Meters.vi"("Units Selector"=w67, "Units"=w94) -> ("Meters"=w95:dbl)  [unwired: 9 in]
        n51 = call "Create_Trajectory_Value_Units_To_Meters.vi"("Units Selector"=w67, "Units"=w84) -> ("Meters"=w85:dbl)  [unwired: 9 in]
        n52 = call "Create_Trajectory_Value_Units_To_Meters.vi"("Units Selector"=w67, "Units"="Region Max Speed (Units/Sec)") -> ("Meters"=w36:dbl)  [unwired: 9 in]
        "Region Max Speed M/Sec" <- w36
        n53 = call "Create_Trajectory_Value_Units_To_Meters.vi"("Units Selector"=w67, "Units"=w79) -> ("Meters"=w80:dbl)  [unwired: 9 in]
        n54 = Reciprocal(x=w102) -> (1/x=w103:dbl)
        n55 = call "Create_Trajectory_Value_Units_To_Meters.vi"("Units Selector"=w67, "Units"=w77) -> ("Meters"=w78:dbl)  [unwired: 9 in]
        n56 = Reciprocal(x=w109) -> (1/x=w106:dbl)
        n57 = call "Create_Trajectory_Value_Units_To_Meters.vi"("Units Selector"=w67, "Units"=w73) -> ("Meters"=w74:dbl)  [unwired: 9 in]
        n58 = call "Create_Trajectory_Value_Units_To_Meters.vi"("Units Selector"=w67, "Units"=w91) -> ("Meters"=w92:dbl)  [unwired: 9 in]
        n59 = call "Create_Trajectory_Value_Units_To_Meters.vi"("Units Selector"=w67, "Units"=w96) -> ("Meters"=w97:dbl)  [unwired: 9 in]
        n60 = call "Create_Trajectory_Value_Units_To_Meters.vi"("Units Selector"=w67, "Units"=w86) -> ("Meters"=w87:dbl)  [unwired: 9 in]
        n61 = local read "MaxAcceleration"() -> (w112:dbl)
        n62 = call "Create_Trajectory_Value_Units_To_Meters.vi"("Units Selector"=w67, "Units"=w81) -> ("Meters"=w82:dbl)  [unwired: 9 in]
        n63 = local read "MaxVelocity"() -> (w113:dbl)
        n64 = local read "Max Cent Accel"() -> (w110:dbl)
        n65 = local read "Track Width"() -> (w111:dbl)
        n66 = call "Create_Trajectory_Value_Units_To_Meters.vi"("Units Selector"=w67, "Units"=w103) -> ("Meters"=w104:dbl)  [unwired: 9 in]
        n67 = call <vilib>:"Translation2d_Create.vi"("Y"=w78, "X"=w76) -> ("TRANSLATION"=w38:T7)  [unwired: 9 in]
        "Rect Reg Bot Left M" <- w38
        n68 = call <vilib>:"Translation2d_Create.vi"("Y"=w74, "X"=w72) -> ("TRANSLATION"=w37:T7)  [unwired: 9 in]
        "Rect Reg Top Right M" <- w37
        n69 = call <vilib>:"Translation2d_Create.vi"("Y"=w92, "X"=w90) -> ("TRANSLATION"=w40:T7)  [unwired: 9 in]
        "Mech Left Rear M" <- w40
        n70 = call <vilib>:"Translation2d_Create.vi"("Y"=w97, "X"=w95) -> ("TRANSLATION"=w39:T7)  [unwired: 9 in]
        "Mech Right Rear M" <- w39
        n71 = call <vilib>:"Translation2d_Create.vi"("Y"=w87, "X"=w85) -> ("TRANSLATION"=w41:T7)  [unwired: 9 in]
        "Mech Right Front M" <- w41
        n72 = call "Create_Trajectory_Value_Units_To_Meters.vi"("Units Selector"=w67, "Units"=w106) -> ("Meters"=w107:dbl)  [unwired: 9 in]
        n73 = call <vilib>:"Translation2d_Create.vi"("Y"=w82, "X"=w80) -> ("TRANSLATION"=w42:T7)  [unwired: 9 in]
        "Mech Left Front M" <- w42
        n74 = Reciprocal(x=w104) -> (1/x=w105:dbl)
        n75 = Reciprocal(x=w107) -> (1/x=w108:dbl)
        n76 = call "Create_Trajectory_Value_Units_To_Meters.vi"("Units Selector"=w67, "Units"=w113) -> ("Meters"=w45:dbl)  [unwired: 9 in]
        "MaxVelocity M/S" <- w45
        n77 = call "Create_Trajectory_Value_Units_To_Meters.vi"("Units Selector"=w67, "Units"=w112) -> ("Meters"=w44:dbl)  [unwired: 9 in]
        "MaxAcceleration M/S^2" <- w44
        n78 = call <vilib>:"SimpleMotorFF_New.vi"("Ka"=w108, "Kv"=w105, "Ks"=w101) -> ("SIMPLE_MOTOR_FF"=w47:T11)  [unwired: 8 in]
        "SIMPLE_MOTOR_FF M" <- w47
        n79 = call "Create_Trajectory_Value_Units_To_Meters.vi"("Units Selector"=w67, "Units"=w110) -> ("Meters"=w46:dbl)  [unwired: 9 in]
        "Max Cent Accel M/S^2" <- w46
        n80 = call "Create_Trajectory_Value_Units_To_Meters.vi"("Units Selector"=w67, "Units"=w111) -> ("Meters"=w43:dbl)  [unwired: 9 in]
        "Track Width M" <- w43
        n81 = local read "Use Rectangular Region\nMax Velocity Constraint"() -> (w53:bool)
        n82 = local read "Use Mecanum \nDrive\nKinematics\nConstraint"() -> (w66:bool)
        n83 = local read "Use Swerve Drive\nKinematics\nConstraint"() -> (w65:bool)
        n84 = local read "Use Diff Drive\nVoltage\nConstraint"() -> (w60:bool)
        n85 = local read "Max Voltage"() -> (w61:dbl)
        n86 = local read "Use Diff Drive\nKinematic\nConstraint"() -> (w63:bool)
        n87 = local read "Use Centripetal\nAcceleration\nConstaint"() -> (w62:bool)
        n88 = local read "Reverse"() -> (w64:bool)
        n89 = call <vilib>:"SwerveKinematics_NewX.vi"("Wheels"=w48) -> ("SWERVE_DRIVE_KINEMATICS"=w49:T17)  [unwired: 10 in]
        n90 = call <vilib>:"TrajectoryConfig_Create.vi"("MaxAcceleration"=w44, "MaxVelocity"=w45) -> ("TRAJECTORY_CONFIG"=w58:T2)  [unwired: 9 in]
        n91 = call <vilib>:"MecaKinematics_New.vi"("RearRight"=w39, "RearLeft"=w40, "FrontRight"=w41, "FrontLeft"=w42) -> ("MECA_DRIVE_KINEMATICS"=w50:T20)  [unwired: 7 in]
        n92 = flat-sequence {
          tunnel: w35 -> [_]
          frame #0 {
            # "Update trajectory..."
            n93 = local read "WayPoints"() -> (w115:T3[])
            n94 = Array Size(array=w115) -> (size(s)=w117:i32)
            n95 = Greater Or Equal?(x=w117, y=2) -> (x >= y?=w114:bool)
            n96 = case shown="True" w114 {
              frame False {
              }
              frame True {
                n97 = property on="Calculate\nTrajectory" class="Bool (strict)"("Val(Sgnl)"=TRUE ("Value (Signaling)")) -> ()  [unwired: 2 in, 2 out]
              }
            }
          }
        }
        n98 = call <vilib>:"TrajectoryConfig_setReversed.vi"("Reversed"=w64, "inTRAJECTORY_CONFIG"=w58) -> ("outTRAJECTORY_CONFIG"=w59:T2)  [unwired: 9 in]
        n99 = call <vilib>:"DiffKinematics_New.vi"("TrackWidth_Meters"=w43) -> ("DIFF_DRIVE_KINEMATICS"=w51:T1)  [unwired: 10 in]
        "DIFF_DRIVE_KINEMATICS" <- w51
        n100 = case shown="True" w63 {
          tunnel: w59 -> [w145 w148]
          tunnel: [w145 w147] -> w54
          tunnel: w51 -> [_ w146]
          frame False {
          }
          frame True {
            n101 = call <vilib>:"TrajectoryConfig_setKinematicsDiffDrive.vi"("DIFF_DRIVE_KINEMATICS"=w146, "inTRAJECTORY_CONFIG"=w148) -> ("outTRAJECTORY_CONFIG"=w147:T2)  [unwired: 9 in]
          }
        }
        n102 = case shown="True" w62 {
          tunnel: w54 -> [w141 w144]
          tunnel: [w141 w143] -> w55
          tunnel: w46 -> [_ w142]
          frame False {
          }
          frame True {
            n103 = call <vilib>:"TrajectoryConfig_setCentripetalAccel.vi"("Max Cent Accel"=w142, "inTRAJECTORY_CONFIG"=w144) -> ("outTRAJECTORY_CONFIG"=w143:T2)  [unwired: 9 in]
          }
        }
        n104 = case shown="True" w60 {
          tunnel: w55 -> [w135 w140]
          tunnel: [w135 w139] -> w56
          tunnel: w61 -> [_ w138]
          tunnel: w47 -> [_ w137]
          tunnel: w51 -> [_ w136]
          frame False {
          }
          frame True {
            n105 = call <vilib>:"TrajectoryConfig_setVoltageDiffDrive.vi"("SIMPLE_MOTOR_FF"=w137, "DIFF_DRIVE_KINEMATICS"=w136, "Max Voltage"=w138, "inTRAJECTORY_CONFIG"=w140) -> ("outTRAJECTORY_CONFIG"=w139:T2)  [unwired: 7 in]
          }
        }
        n106 = case shown="True" w65 {
          tunnel: [w131 w134] -> w57
          tunnel: w56 -> [w131 w133]
          tunnel: w49 -> [_ w132]
          frame False {
          }
          frame True {
            n107 = call <vilib>:"TrajectoryConfig_setKinematicsSwerveDrive.vi"("SWERVE_DRIVE_KINEMATICS"=w132, "inTRAJECTORY_CONFIG"=w133) -> ("outTRAJECTORY_CONFIG"=w134:T2)  [unwired: 9 in]
          }
        }
        n108 = case shown="True" w66 {
          tunnel: [w127 w130] -> w52
          tunnel: w57 -> [w127 w129]
          tunnel: w50 -> [_ w128]
          frame False {
          }
          frame True {
            n109 = call <vilib>:"TrajectoryConfig_setKinematicsMecanumDrive.vi"("MECA_DRIVE_KINEMATICS"=w128, "inTRAJECTORY_CONFIG"=w129) -> ("outTRAJECTORY_CONFIG"=w130:T2)  [unwired: 9 in]
          }
        }
        n110 = case shown="True" w53 {
          tunnel: w52 -> [w119 w125]
          tunnel: [w119 w124] -> w35
          tunnel: w38 -> [_ w123]
          tunnel: w37 -> [_ w122]
          tunnel: w36 -> [_ w120]
          frame False {
          }
          frame True {
            n111 = call <vilib>:"MaxVelocityConstraint_New.vi"("Maximum Velocity"=w120) -> ("MAX_VELOCITY_CONSTRAINT"=w121:T21)  [unwired: 10 in]
            n112 = call <vilib>:"RectRegionConstraint_New.vi"("Constraint Data Cluster"=w121, "TopRightPoint"=w122, "BottomLeftPoint"=w123) -> ("RECT_REGION_CONSTRAINT"=w126:T22)  [unwired: 8 in]
            n113 = call <vilib>:"TrajectoryConfig_AddConstraint.vi"("Constraint"=w126, "inTRAJECTORY_CONFIG"=w125) -> ("outTRAJECTORY_CONFIG"=w124:T2)  [unwired: 9 in]
          }
        }
        "outTRAJECTORY_CONFIG" <- w35
      }
      event "UseWeights", "Spline Type": Value Change {
        n114 = event-data() -> ()  [unwired: 1 in, 6 out]
        n115 = local read "WayPoints_M"() -> (w159:T3[])
        n116 = Array Size(array=w159) -> (size(s)=w158:i32)
        n117 = Greater Or Equal?(x=w158, y=2) -> (x >= y?=w156:bool)
        n118 = case shown="True" w156 {
          frame False {
          }
          frame True {
            n119 = property on="Calculate\nTrajectory" class="Bool (strict)"("Val(Sgnl)"=TRUE ("Value (Signaling)")) -> ()  [unwired: 2 in, 2 out]
          }
        }
      }
      event "Reverse": Value Change {
        # "Go through all the waypoints and add 180 degrees to their heading..."
        n120 = event-data() -> ()  [unwired: 1 in, 6 out]
        n121 = local read "WayPoints"() -> (w163:T3[])
        n122 = for {
          tunnel: w163 -> [w169] mode=indexing
          tunnel: [w168] -> w162 mode=indexing
          n123 = in-place {
            n124 = in-place-cluster #3(w169) -> ("ANGLE"=w175:dbl)
            n125 = Add(x=w175, y=180.0) -> (x+y=w171:dbl)
            n126 = call <vilib>:"MathUtil_InputModulus.vi"("Maximum_Input"=180.0, "Minimum_Input"=-180.0, "Input"=w171) -> ("modulus"=w170:dbl)  [unwired: 8 in]
            n127 = in-place-cluster #3("ANGLE"=w170) -> (w168:T3)
          }
        }
        n128 = local read "Units Selector"() -> (w161:T10)
        n129 = call "Create_Trajectory_All_WP_Units_To_Meters.vi"("Units Selector"=w161, "WayPoints"=w162) -> ("Array"=w164:T3[])  [unwired: 9 in]
        n130 = local write "WayPoints"(w162) -> ()
        n131 = local write "WayPoints_M"(w164) -> ()
        n132 = Array Size(array=w164) -> (size(s)=w167:i32)
        n133 = Greater Or Equal?(x=w167, y=2) -> (x >= y?=w165:bool)
        n134 = case shown="True" w165 {
          frame False {
          }
          frame True {
            n135 = property on="Calculate\nTrajectory" class="Bool (strict)"("Val(Sgnl)"=TRUE ("Value (Signaling)")) -> ()  [unwired: 2 in, 2 out]
          }
        }
      }
      event "End Program": Value Change {
        n136 = event-data() -> ("NewVal"=w177:bool)  [unwired: 1 in, 5 out]
        n137 = case shown="True" w177 {
          frame False {
          }
          frame True {
            # "The code doesn't seem to work\ninside the event handler...."
            n138 = local write "Terminate"(TRUE ("Terminate")) -> ()
          }
        }
      }
      event "WriteJSONFile": Value Change {
        n139 = event-data() -> ("NewVal"=w179:bool)  [unwired: 1 in, 5 out]
        n140 = local read "Trajectory\nCompleted\nError Free"() -> (w181:bool)
        n141 = And(x=w179, y=w181) -> (x .and. y?=w180:bool)
        n142 = case shown="True" w180 {
          frame False {
          }
          frame True {
            n143 = local read "Trajectory Type"() -> (w192:enum32{"Radio Selection 1", "Radio Selection 2"})
            n144 = local read "TRAJECTORY"() -> (w193:T4)
            n145 = case shown="\"Radio Selection 1\", Default" w192 {
              tunnel: w193 -> [w209 w211]
              tunnel: [w208 w211] -> w190
              tunnel: [TRUE FALSE] -> _
              frame "Radio Selection 1", Default {
                # "Relative"
                n146 = call <vilib>:"Util_Trajectory_Absolute_To_Relative.vi"("absTRAJECTORY"=w209) -> ("outputRelativeTRAJECTORY"=w208:T4)  [unwired: 10 in]
              }
              frame "Radio Selection 2" {
                # "Absolute"
              }
            }
            n147 = Empty String/Path?(string/path="Trajectory JSON File Name") -> (empty?=w184:bool)
            n148 = case shown="False" w184 {
              tunnel: "Trajectory JSON File Name" -> [w196 w198]
              tunnel: [w194 w198] -> w182
              frame False {
                n149 = call <vilib>:"FileUtil_DefaultDir.vi"("Path in"=w196) -> ("Path Out"=w195:path)  [unwired: 10 in]
                n150 = call <vilib>:"FileUtil_AddExt.vi"("Extension"="json", "Path in"=w195) -> ("Path out"=w194:path)  [unwired: 9 in]
                n151 = local write "Trajectory JSON File Name"(w194) -> ()
              }
              frame True {
                # "empty -- pass \nthrough, will\ncause dialog box."
              }
            }
            n152 = call <vilib>:"Trajectory_GetStates.vi"("TRAJECTORY"=w190) -> ("States"=w191:T5[])  [unwired: 10 in]
            n153 = call "Create_Trajectory_Traj_Meters_To_PW_Units.vi"("States in_M"=w191, "PathWeaver Length Units"="PathWeaver Length Units") -> ("States out_UNITS"=w189:T5[])  [unwired: 9 in]
            n154 = call <vilib>:"Trajectory_New.vi"("TRAJ_STATES"=w189) -> ("TRAJECTORY"=w188:T4)  [unwired: 10 in]
            n155 = Path To String(path=w182) -> (string=w185:string)
            n156 = call <vilib>:"TrajectoryUtil_toPathWeaverJSON.vi"("inTRAJECTORY"=w188, "FileName"=w185) -> ("error out"=w186:errorcluster)  [unwired: 8 in, 1 out]
            n157 = case shown="Error .." w186 {
              selector: w186 -> [_ w203]
              tunnel: w185 -> [w201 _]
              frame No Error {
                n158 = Concatenate Strings("Trajectory JSON file, " ("message"), w201, ", saved." ("string")) -> (w199:string)
                n159 = One Button Dialog(message=w199) -> ()  [unwired: 1 in, 1 out]
              }
              frame Error {
                w204 = T24 1 items=["no dialog", "OK message", "continue or stop message", "OK message + warnings", "continue/stop + warnings"] ("type of dialog (OK msg:1)")
                n160 = Unbundle By Name(w203) -> ("code"=w206:i32, "source"=w205:string)
                n161 = call <vilib>:"Simple Error Handler.vi"("error code (no error:0)"=w206, "error source (\" \")"=w205, "type of dialog (OK msg:1)"=w204, "error in (no error)"=w203) -> ()  [unwired: 1 in, 5 out]
              }
            }
          }
        }
      }
      event "ReadConfigFile": Value Change {
        n162 = event-data() -> ("NewVal"=w212:bool)  [unwired: 1 in, 5 out]
        n163 = case shown="True" w212 {
          frame False {
          }
          frame True {
            # "#TODO Fix read file for\nV5 variant issue."
            # "#TODO Need to clear and rebuild cursors!!!"
            # "Read\nFile"
            # "Read config from trajectory File"
            n164 = Empty String/Path?(string/path="Read Config File Name") -> (empty?=w216:bool)
            n165 = case shown="False" w216 {
              tunnel: "Read Config File Name" -> [w222 w224]
              tunnel: [w220 w224] -> w214
              frame False {
                n166 = call <vilib>:"FileUtil_DefaultDir.vi"("Path in"=w222) -> ("Path Out"=w221:path)  [unwired: 10 in]
                n167 = call <vilib>:"FileUtil_AddExt.vi"("Extension"="xml", "Path in"=w221) -> ("Path out"=w220:path)  [unwired: 9 in]
              }
              frame True {
                # "empty -- pass \nthrough, will\ncause dialog box."
              }
            }
            n168 = call-poly <vilib>:"Read From XML File.vi"("XML File Path"=w214) -> ("error out"=w218:errorcluster, "XML Elements"=w217:string, "XML File Path(duplicate)"=w213:path)  [unwired: 8 in]
            n169 = local write "Read Config File Name"(w213) -> ()
            n170 = case shown="No Error" w218 {
              tunnel: w217 -> [w228 _]
              tunnel: w218 -> [w227 w353]
              tunnel: [w230 "" ("Write Config File Comment")] -> w219
              frame No Error {
                # "parse\nXML"
                # "A little bit of a \nkludge to read \nboth v2 and v1\nfile formats...."
                n171 = local read "Units Selector"() -> (w225:T10)
                n172 = call "Create_Trajectory_Config_Parse_V1_V2_V3.vi"("error in (no error)"=w227, "Units Selector"=w225, "XML Elements"=w228) -> ("error out"=w229:errorcluster, "TrajCreateConfig"=w226:T16)  [unwired: 7 in]
                n173 = case shown="No Error" w229 {
                  tunnel: w226 -> [w236 _]
                  tunnel: [w235 "" ("Write Config File Comment")] -> w230
                  tunnel: w229 -> [w234 w350]
                  frame No Error {
                    # "Create and draw \ntrajectory."
                    n174 = flat-sequence {
                      tunnel: w236 -> [w270]
                      tunnel: [w322] -> w235
                      tunnel: w234 -> [_]
                      tunnel: [w271] -> w231
                      frame #0 {
                        # "Update cursors..."
                        # "Field is always\ninches..."
                        # "Write to local\nuser controls"
                        # "not used"
                        # "not used"
                        n175 = Unbundle By Name(w270) -> ("Write Config File Name"=w281:path, "Write Config File Comment"=w322:string, "WayPoints"=w276:T3[], "TRAJECTORY_CONFIG"=w258:T2, "IsCubic"=w277:bool, "Units Selector"=w242:T10, "UseWeights"=w279:bool)
                        n176 = call "Create_Trajectory_Parse_RectRegion_Constraint.vi"("inTRAJECTORY_CONFIG"=w258) -> ("Constraint Exists"=w249:bool, "Max Speed"=w246:dbl, "BottomLeftPoint"=w247:T7, "TopRightPoint"=w248:T7)  [unwired: 7 in]
                        n177 = Unbundle By Name(w270) -> ("FieldName"=w269:string)
                        n178 = Unbundle By Name(w258) -> ("MaxVelocity"=w330:dbl, "Max Acceleration"=w329:dbl, "Reversed"=w328:bool)  [unwired: 2 out]
                        n179 = call <vilib>:"TrajectoryConfig_GetKinematicsDiffDriveContraint.vi"("inTRAJECTORY_CONFIG"=w258) -> ("Constraint Exists"=w265:bool, "Diff Drive Kinematics Constraint"=w259:T25)  [unwired: 9 in]
                        n180 = call <vilib>:"TrajectoryConfig_GetCentripetalAccelConstraint.vi"("inTRAJECTORY_CONFIG"=w258) -> ("Constraint Exists"=w264:bool, "Centripital Accleration Constraint"=w268:T26)  [unwired: 9 in]
                        n181 = call <vilib>:"TrajectoryConfig_GetVoltageDiffDriveConstraint.vi"("inTRAJECTORY_CONFIG"=w258) -> ("Constraint Exists"=w263:bool, "Differential Drive Voltage Constraint"=w267:T27)  [unwired: 9 in]
                        n182 = call <vilib>:"TrajectoryConfig_GetKinematicsMecanumDriveConstraint.vi"("inTRAJECTORY_CONFIG"=w258) -> ("Constraint Exists"=w261:bool, "Mecanum Drive Kinematics Constraint"=w266:T28)  [unwired: 9 in]
                        n183 = Unbundle By Name(w266) -> ("MECA_DRIVE_KINEMATICS.FrontLeft"=w298:T7, "MECA_DRIVE_KINEMATICS.FrontRight"=w299:T7, "MECA_DRIVE_KINEMATICS.RearLeft"=w300:T7, "MECA_DRIVE_KINEMATICS.RearRight"=w301:T7)
                        n184 = call <vilib>:"TrajectoryConfig_GetKinematicsSwerveDriveConstraint.vi"("inTRAJECTORY_CONFIG"=w258) -> ("Constraint Exists"=w260:bool, "Swerver Drive Kinematics Constraint"=w262:T29)  [unwired: 9 in]
                        n185 = Unbundle By Name(w259) -> ("DIFF_DRIVE_KINEMATICS.TrackWidth_Meters"=w326:dbl)
                        n186 = Unbundle By Name(w268) -> ("Max Cent Accel"=w324:dbl)
                        n187 = Unbundle By Name(w267) -> ("Max Voltage"=w323:dbl, "SIMPLE_MOTOR_FF"=w284:T11)
                        n188 = Unbundle By Name(w262) -> ("SwerveKinematics.Modules"=w318:T7[])
                        n189 = property on="Field Selector" class="CmbBox"("Val(Sgnl)"=w269) -> ()  [unwired: 2 in, 2 out]
                        n190 = call <vilib>:"Translation2d_GetXY.vi"("In Translation"=w248) -> ("Y"=w255:dbl, "X"=w257:dbl)  [unwired: 9 in]
                        n191 = call <vilib>:"Translation2d_GetXY.vi"("In Translation"=w247) -> ("Y"=w251:dbl, "X"=w253:dbl)  [unwired: 9 in]
                        n192 = Unbundle By Name(w284) -> ("Ks"=w293:dbl, "Kv"=w292:dbl, "Ka"=w285:dbl)
                        n193 = call "Create_Trajectory_Value_Meters_To_Units.vi"("Units Selector"=w242, "Meters"=w257) -> ("Units"=w256:dbl)  [unwired: 9 in]
                        n194 = call "Create_Trajectory_Value_Meters_To_Units.vi"("Units Selector"=w242, "Meters"=w253) -> ("Units"=w252:dbl)  [unwired: 9 in]
                        n195 = call "Create_Trajectory_Value_Meters_To_Units.vi"("Units Selector"=w242, "Meters"=w255) -> ("Units"=w254:dbl)  [unwired: 9 in]
                        n196 = call "Create_Trajectory_Value_Meters_To_Units.vi"("Units Selector"=w242, "Meters"=w251) -> ("Units"=w250:dbl)  [unwired: 9 in]
                        n197 = call "Create_Trajectory_Value_Meters_To_Units.vi"("Units Selector"=w242, "Meters"=w246) -> ("Units"=w245:dbl)  [unwired: 9 in]
                        n198 = call "Create_Trajectory_All_WP_Meters_To_Units.vi"("Units Selector"=TrajCreateUnitsENUM."Inches", "WayPoints_M"=w276) -> ("outWayPoints_UNITS"=w275:T3[])  [unwired: 9 in]
                        n199 = call "Create_Trajectory_All_WP_Meters_To_Units.vi"("Units Selector"=w242, "WayPoints_M"=w276) -> ("outWayPoints_UNITS"=w272:T3[])  [unwired: 9 in]
                        n200 = case shown="True" w277 {
                          tunnel: [enum32{"Radio Selection 1", "Radio Selection 2"}."Radio Selection 2" ("Spline Type") enum32{"Radio Selection 1", "Radio Selection 2"}."Radio Selection 1" ("Spline Type")] -> w333
                          frame False {
                          }
                          frame True {
                          }
                        }
                        n201 = Reciprocal(x=w292) -> (1/x=w291:dbl)
                        n202 = Reciprocal(x=w285) -> (1/x=w288:dbl)
                        n203 = call "ChangeFileExtension.vi"("NewExtenion"=".json", "In FileName"=w281) -> ("Out FileName"=w280:path)  [unwired: 9 in]
                        n204 = call "ChangeFileExtension.vi"("NewExtenion"=".csv", "In FileName"=w281) -> ("Out FileName"=w321:path)  [unwired: 9 in]
                        n205 = call <vilib>:"Translation2d_GetXY.vi"("In Translation"=w298) -> ("Y"=w315:dbl, "X"=w317:dbl)  [unwired: 9 in]
                        n206 = call <vilib>:"Translation2d_Create.vi"("Y"=w254, "X"=w256) -> ("TRANSLATION"=w244:T7)  [unwired: 9 in]
                        n207 = call <vilib>:"Translation2d_Create.vi"("Y"=w250, "X"=w252) -> ("TRANSLATION"=w243:T7)  [unwired: 9 in]
                        n208 = call <vilib>:"Translation2d_GetXY.vi"("In Translation"=w299) -> ("Y"=w311:dbl, "X"=w313:dbl)  [unwired: 9 in]
                        n209 = call <vilib>:"Translation2d_GetXY.vi"("In Translation"=w300) -> ("Y"=w307:dbl, "X"=w309:dbl)  [unwired: 9 in]
                        n210 = for {
                          tunnel: w318 -> [w341] mode=indexing
                          tunnel: [w340] -> w319 mode=indexing
                          tunnel: w242 -> [w339]
                          n211 = call <vilib>:"Translation2d_GetXY.vi"("In Translation"=w341) -> ("Y"=w343:dbl, "X"=w345:dbl)  [unwired: 9 in]
                          n212 = call "Create_Trajectory_Value_Meters_To_Units.vi"("Units Selector"=w339, "Meters"=w345) -> ("Units"=w344:dbl)  [unwired: 9 in]
                          n213 = call "Create_Trajectory_Value_Meters_To_Units.vi"("Units Selector"=w339, "Meters"=w343) -> ("Units"=w342:dbl)  [unwired: 9 in]
                          n214 = call <vilib>:"Translation2d_Create.vi"("Y"=w342, "X"=w344) -> ("TRANSLATION"=w340:T7)  [unwired: 9 in]
                        }
                        n215 = call <vilib>:"Translation2d_GetXY.vi"("In Translation"=w301) -> ("Y"=w303:dbl, "X"=w305:dbl)  [unwired: 9 in]
                        n216 = call "Create_Trajectory_Value_Meters_To_Units.vi"("Units Selector"=w242, "Meters"=w291) -> ("Units"=w290:dbl)  [unwired: 9 in]
                        n217 = local write "Region Max Speed (Units/Sec)"(w245) -> ()
                        n218 = local write "WayPoints"(w272) -> ()
                        n219 = local write "Use Rectangular Region\nMax Velocity Constraint"(w249) -> ()
                        n220 = for {
                          tunnel: w275 -> [w337] mode=indexing
                          tunnel: [w334] -> w273 mode=indexing
                          n221 = Unbundle By Name(w337) -> ("X"=w336:dbl, "Y"=w335:dbl)
                          n222 = Bundle By Name(cluster=T15 {"Name"="Cursor", "Color"=915580, "Style"=4, "Point Style"=2, "Name Visible"=FALSE, "Allow Drag"=TRUE, "Cursor Mode"=0, "Plot"=0, "Index"=0, "Position"={"X"=315.0, "Y"=162.0}, "X Scale"=0, "Y Scale"=0, "Watch Plots"=[], "Watch All Plots"=FALSE, "Plot Area"=0, "Label Offset"={"X"=0.0, "Y"=0.0}} ("new element/subarray"), "Position.X"=w336, "Position.Y"=w335) -> (w334:T15)
                        }
                        n223 = call "Create_Trajectory_Value_Meters_To_Units.vi"("Units Selector"=w242, "Meters"=w288) -> ("Units"=w287:dbl)  [unwired: 9 in]
                        n224 = local write "outTRAJECTORY_CONFIG"(w258) -> ()
                        n225 = local write "Rect Reg Top Right"(w244) -> ()
                        n226 = local write "REct Reg Bot Left"(w243) -> ()
                        n227 = local write "Units Selector"(w242) -> ()
                        n228 = local write "WayPoints_M"(w276) -> ()
                        n229 = local write "Trajectory JSON File Name"(w280) -> ()
                        n230 = local write "Trajectory CSV File Name"(w321) -> ()
                        n231 = call "Create_Trajectory_Value_Meters_To_Units.vi"("Units Selector"=w242, "Meters"=w317) -> ("Units"=w316:dbl)  [unwired: 9 in]
                        n232 = local write "Trajectory\nCompleted\nError Free"(FALSE ("Trajectory\nCompleted\nError Free")) -> ()
                        n233 = call "Create_Trajectory_Value_Meters_To_Units.vi"("Units Selector"=w242, "Meters"=w330) -> ("Units"=w331:dbl)  [unwired: 9 in]
                        n234 = call "Create_Trajectory_Value_Meters_To_Units.vi"("Units Selector"=w242, "Meters"=w329) -> ("Units"=w332:dbl)  [unwired: 9 in]
                        n235 = call "Create_Trajectory_Value_Meters_To_Units.vi"("Units Selector"=w242, "Meters"=w313) -> ("Units"=w312:dbl)  [unwired: 9 in]
                        n236 = local write "IsCubic"(w277) -> ()
                        n237 = local write "UseWeights"(w279) -> ()
                        n238 = local write "Write Config File Name"(w281) -> ()
                        n239 = local write "Write Config File Comment"(w322) -> ()
                        n240 = local write "Trajectory File Comment"(w322) -> ()
                        n241 = call "Create_Trajectory_Value_Meters_To_Units.vi"("Units Selector"=w242, "Meters"=w309) -> ("Units"=w308:dbl)  [unwired: 9 in]
                        n242 = Reciprocal(x=w290) -> (1/x=w289:dbl)
                        n243 = call "Create_Trajectory_Value_Meters_To_Units.vi"("Units Selector"=w242, "Meters"=w305) -> ("Units"=w304:dbl)  [unwired: 9 in]
                        n244 = Reciprocal(x=w287) -> (1/x=w286:dbl)
                        n245 = call "Create_Trajectory_Value_Meters_To_Units.vi"("Units Selector"=w242, "Meters"=w315) -> ("Units"=w314:dbl)  [unwired: 9 in]
                        n246 = call "Create_Trajectory_Value_Meters_To_Units.vi"("Units Selector"=w242, "Meters"=w311) -> ("Units"=w310:dbl)  [unwired: 9 in]
                        n247 = Array Size(array=w272) -> (size(s)=w271:i32)
                        n248 = local write "Use Mecanum \nDrive\nKinematics\nConstraint"(w261) -> ()
                        n249 = call "Create_Trajectory_Value_Meters_To_Units.vi"("Units Selector"=w242, "Meters"=w307) -> ("Units"=w306:dbl)  [unwired: 9 in]
                        n250 = call "Create_Trajectory_Value_Meters_To_Units.vi"("Units Selector"=w242, "Meters"=w303) -> ("Units"=w302:dbl)  [unwired: 9 in]
                        n251 = call "Create_Trajectory_Value_Meters_To_Units.vi"("Units Selector"=w242, "Meters"=w326) -> ("Units"=w327:dbl)  [unwired: 9 in]
                        n252 = call "Create_Trajectory_Value_Meters_To_Units.vi"("Units Selector"=w242, "Meters"=w324) -> ("Units"=w325:dbl)  [unwired: 9 in]
                        n253 = local write "Use Swerve Drive\nKinematics\nConstraint"(w260) -> ()
                        n254 = local write "Use Centripetal\nAcceleration\nConstaint"(w264) -> ()
                        n255 = call <vilib>:"SimpleMotorFF_New.vi"("Ka"=w286, "Kv"=w289, "Ks"=w293) -> ("SIMPLE_MOTOR_FF"=w283:T11)  [unwired: 8 in]
                        n256 = local write "Use Diff Drive\nKinematic\nConstraint"(w265) -> ()
                        n257 = local write "MaxVelocity"(w331) -> ()
                        n258 = local write "MaxAcceleration"(w332) -> ()
                        n259 = local write "Spline Type"(w333) -> ()
                        n260 = call <vilib>:"Translation2d_Create.vi"("Y"=w314, "X"=w316) -> ("TRANSLATION"=w297:T7)  [unwired: 9 in]
                        n261 = local write "Reverse"(w328) -> ()
                        n262 = local write "Use Diff Drive\nVoltage\nConstraint"(w263) -> ()
                        n263 = call <vilib>:"Translation2d_Create.vi"("Y"=w310, "X"=w312) -> ("TRANSLATION"=w296:T7)  [unwired: 9 in]
                        n264 = call <vilib>:"Translation2d_Create.vi"("Y"=w306, "X"=w308) -> ("TRANSLATION"=w295:T7)  [unwired: 9 in]
                        n265 = call <vilib>:"Translation2d_Create.vi"("Y"=w302, "X"=w304) -> ("TRANSLATION"=w294:T7)  [unwired: 9 in]
                        n266 = local write "Max Cent Accel"(w325) -> ()
                        n267 = local write "Track Width"(w327) -> ()
                        n268 = local write "SIMPLE_MOTOR_FF"(w283) -> ()
                        n269 = local write "Mech Left Front"(w297) -> ()
                        n270 = local write "Mech Right Front"(w296) -> ()
                        n271 = local write "Max Voltage"(w323) -> ()
                        n272 = local write "Mech Right Rear"(w294) -> ()
                        n273 = local write "Mech Left Rear"(w295) -> ()
                        n274 = local write "Swerve Wheels"(w319) -> ()
                        n275 = property on="Position" class="XYGraph (strict)"("CrsrList"=w273) -> ()  [unwired: 2 in, 2 out]
                      }
                    }
                    n276 = Greater Or Equal?(x=w231, y=2) -> (x >= y?=w232:bool)
                    n277 = flat-sequence {
                      tunnel: w231 -> [_]
                      frame #0 {
                        n278 = local read "Update\nConfig"() -> (w238:bool)
                        n279 = Not(x=w238) -> (.not. x?=w237:bool)
                        n280 = property on="Update\nConfig" class="Bool (strict)"("Val(Sgnl)"=w237) -> ()  [unwired: 2 in, 2 out]
                        n281 = One Button Dialog(message="Configuration file\nread without error.") -> ()  [unwired: 1 in, 1 out]
                      }
                    }
                    n282 = case shown="True" w232 {
                      frame False {
                        n283 = local write "TRAJECTORY"(T4 {"TotalTImeSecs"=0.0, "States"=[]} ("TRAJECTORY")) -> ()
                      }
                      frame True {
                        n284 = property on="Calculate\nTrajectory" class="Bool (strict)"("Val(Sgnl)"=TRUE ("Value (Signaling)")) -> ()  [unwired: 2 in, 2 out]
                      }
                    }
                  }
                  frame Error {
                    w348 = T24 1 items=["no dialog", "OK message", "continue or stop message", "OK message + warnings", "continue/stop + warnings"] ("type of dialog (OK msg:1)")
                    n285 = Unbundle By Name(w350) -> ("code"=w351:i32, "source"=w349:string)
                    n286 = call <vilib>:"Simple Error Handler.vi"("error code (no error:0)"=w351, "error source (\" \")"=w349, "type of dialog (OK msg:1)"=w348, "error in (no error)"=w350) -> ()  [unwired: 1 in, 5 out]
                  }
                }
              }
              frame Error {
                w354 = T24 1 items=["no dialog", "OK message", "continue or stop message", "OK message + warnings", "continue/stop + warnings"] ("type of dialog (OK msg:1)")
                n287 = Unbundle By Name(w353) -> ("code"=w356:i32, "source"=w355:string)
                n288 = call <vilib>:"Simple Error Handler.vi"("error code (no error:0)"=w356, "error source (\" \")"=w355, "type of dialog (OK msg:1)"=w354, "error in (no error)"=w353) -> ()  [unwired: 1 in, 5 out]
              }
            }
            "Read Config File Comment" <- w219
          }
        }
      }
      event "WriteConfigFile": Value Change {
        n289 = event-data() -> ("NewVal"=w359:bool)  [unwired: 1 in, 5 out]
        n290 = local read "Trajectory\nCompleted\nError Free"() -> (w360:bool)
        n291 = And(x=w359, y=w360) -> (x .and. y?=w358:bool)
        n292 = case shown="True" w358 {
          frame False {
          }
          frame True {
            # "Convert\ninternal\nto V5"
            # "write xml\nfile"
            # "convert\nto xml\nstring"
            n293 = local read "outTRAJECTORY_CONFIG"() -> (w365:T2)
            n294 = local read "Field Selector"() -> (w368:string)
            n295 = local read "WayPoints_M"() -> (w374:T3[])
            n296 = local read "UseWeights"() -> (w375:bool)
            n297 = local read "IsCubic"() -> (w377:bool)
            n298 = local read "Units Selector"() -> (w376:T10)
            n299 = Empty String/Path?(string/path="Write Config File Name") -> (empty?=w363:bool)
            n300 = case shown="False" w363 {
              tunnel: "Write Config File Name" -> [w380 w382]
              tunnel: [w378 w382] -> w361
              frame False {
                n301 = call <vilib>:"FileUtil_DefaultDir.vi"("Path in"=w380) -> ("Path Out"=w379:path)  [unwired: 10 in]
                n302 = call <vilib>:"FileUtil_AddExt.vi"("Extension"="xml", "Path in"=w379) -> ("Path out"=w378:path)  [unwired: 9 in]
                n303 = local write "Write Config File Name"(w378) -> ()
              }
              frame True {
                # "empty -- pass \nthrough, will\ncause dialog box."
              }
            }
            n304 = Bundle By Name(cluster=T16 {"Write Config File Name"=path "", "Write Config File Comment"="", "WayPoints"=[], "TRAJECTORY_CONFIG"={"MaxVelocity"=0.0, "Max Acceleration"=0.0, "StartVelocity"=0.0, "End Velocity"=0.0, "Reversed"=FALSE, "Constraints"=[]}, "IsCubic"=FALSE, "Units Selector"=enum."Inches", "UseWeights"=FALSE, "FieldName"=""} ("TrajCreateConfig"), "Write Config File Name"=w361, "Write Config File Comment"="Write Config File Comment", "WayPoints"=w374, "TRAJECTORY_CONFIG"=w365, "IsCubic"=w377, "Units Selector"=w376, "UseWeights"=w375, "FieldName"=w368) -> (w367:T16)
            n305 = local write "Trajectory File Comment"("Write Config File Comment") -> ()
            n306 = call "Creat_Traj_Config_Convert_V_internal_To_V5.vi"("TrajCreateConfig V_Internal"=w367) -> ("TrajCreateConfig V5"=w366:T30)  [unwired: 10 in]
            n307 = Flatten To XML(anything=w366) -> (xml string=w371:string)
            n308 = call-poly <vilib>:"Write to XML File.vi"("Standalone? (T)"=TRUE, "XML Input"=w371, "XML File Path"=w361) -> ("error out"=w372:errorcluster, "XML File Path(duplicate)"=w364:path)  [unwired: 6 in, 1 out]
            n309 = case shown="No Error" w372 {
              selector: w372 -> [_ w388]
              tunnel: w364 -> [w383 _]
              frame No Error {
                n310 = Path To String(path=w383) -> (string=w384:string)
                n311 = Concatenate Strings("Trajectory config XML  file, " ("message"), w384, ", saved." ("string")) -> (w385:string)
                n312 = One Button Dialog(message=w385) -> ()  [unwired: 1 in, 1 out]
              }
              frame Error {
                w389 = T24 1 items=["no dialog", "OK message", "continue or stop message", "OK message + warnings", "continue/stop + warnings"] ("type of dialog (OK msg:1)")
                n313 = Unbundle By Name(w388) -> ("code"=w391:i32, "source"=w390:string)
                n314 = call <vilib>:"Simple Error Handler.vi"("error code (no error:0)"=w391, "error source (\" \")"=w390, "type of dialog (OK msg:1)"=w389, "error in (no error)"=w388) -> ()  [unwired: 1 in, 5 out]
              }
            }
          }
        }
      }
      event "WriteTrajFile": Value Change {
        n315 = event-data() -> ("NewVal"=w393:bool)  [unwired: 1 in, 5 out]
        n316 = local read "Trajectory\nCompleted\nError Free"() -> (w394:bool)
        n317 = And(x=w393, y=w394) -> (x .and. y?=w392:bool)
        n318 = case shown="True" w392 {
          frame False {
          }
          frame True {
            n319 = local read "UseWeights"() -> (w406:bool)
            n320 = local read "outTRAJECTORY_CONFIG"() -> (w405:T2)
            n321 = local read "TRAJECTORY"() -> (w404:T4)
            n322 = local read "WayPoints_M"() -> (w403:T3[])
            n323 = local read "IsCubic"() -> (w407:bool)
            n324 = Empty String/Path?(string/path="Trajectory CSV File Name") -> (empty?=w397:bool)
            n325 = case shown="False" w397 {
              tunnel: "Trajectory CSV File Name" -> [w410 w412]
              tunnel: [w408 w412] -> w395
              frame False {
                n326 = call <vilib>:"FileUtil_DefaultDir.vi"("Path in"=w410) -> ("Path Out"=w409:path)  [unwired: 10 in]
                n327 = call <vilib>:"FileUtil_AddExt.vi"("Extension"="csv", "Path in"=w409) -> ("Path out"=w408:path)  [unwired: 9 in]
                n328 = local write "Trajectory CSV File Name"(w408) -> ()
              }
              frame True {
                # "empty -- pass \nthrough, will\ncause dialog box."
              }
            }
            n329 = case shown="\"Radio Selection 1\", Default" "Trajectory Type" {
              tunnel: w404 -> [w424 w426]
              tunnel: [w423 w426] -> w398
              tunnel: [TRUE FALSE] -> w400
              frame "Radio Selection 1", Default {
                # "Relative"
                n330 = call <vilib>:"Util_Trajectory_Absolute_To_Relative.vi"("absTRAJECTORY"=w424) -> ("outputRelativeTRAJECTORY"=w423:T4)  [unwired: 10 in]
              }
              frame "Radio Selection 2" {
                # "Absolute"
              }
            }
            n331 = call <vilib>:"Util_Trajectory_WriteFile.vi"("Trajectory is Cubic"=w407, "UseWeights"=w406, "Trajectory Is Relative"=w400, "TRAJECTORY_CONFIG"=w405, "UtilityWayPoints"=w403, "TRAJECTORY"=w398, "Comment"="Trajectory File Comment", "Trajectory File Name"=w395) -> ("error out"=w399:errorcluster)  [unwired: 3 in]
            n332 = case shown="No Error" w399 {
              selector: w399 -> [_ w418]
              tunnel: w395 -> [w414 _]
              frame No Error {
                n333 = Path To String(path=w414) -> (string=w413:string)
                n334 = Concatenate Strings("Trajectory CSV file, " ("message"), w413, ", saved." ("string")) -> (w415:string)
                n335 = One Button Dialog(message=w415) -> ()  [unwired: 1 in, 1 out]
              }
              frame Error {
                w419 = T24 1 items=["no dialog", "OK message", "continue or stop message", "OK message + warnings", "continue/stop + warnings"] ("type of dialog (OK msg:1)")
                n336 = Unbundle By Name(w418) -> ("code"=w421:i32, "source"=w420:string)
                n337 = call <vilib>:"Simple Error Handler.vi"("error code (no error:0)"=w421, "error source (\" \")"=w420, "type of dialog (OK msg:1)"=w419, "error in (no error)"=w418) -> ()  [unwired: 1 in, 5 out]
              }
            }
            n338 = local write "Write Config File Comment"("Trajectory File Comment") -> ()
          }
        }
      }
      event "Field Selector": Value Change {
        n339 = event-data() -> ("NewVal"=w428:string)  [unwired: 1 in, 5 out]
        n340 = local read "FIeldSelectorHasItems"() -> (w427:bool)
        n341 = case shown="True" w427 {
          tunnel: w428 -> [_ w432]
          frame False {
          }
          frame True {
            w429 = 27.0  # Field Y Ft
            w430 = 58.0  # Field X Ft
            n342 = control-ref of="2D Picture"() -> (w433:refnum<vi>)
            n343 = call <vilib>:"FieldDisp_Field_Disp.vi"("Field X Ft"=w430, "Field Y Ft"=w429, "Field Selector"=w432, "Picture in"=w433) -> ("error out"=w431:errorcluster)  [unwired: 7 in]
            n344 = case shown="Error .." w431 {
              frame Error {
                n345 = One Button Dialog(message="The field_picture file could not be read.  Execution will continue normally with a blank playing field.") -> ()  [unwired: 1 in, 1 out]
              }
              frame No Error {
              }
            }
          }
        }
      }
      event "Calculate\nTrajectory": Value Change {
        n346 = event-data() -> ("NewVal"=w435:bool)  [unwired: 1 in, 5 out]
        n347 = case shown="True" w435 {
          frame False {
          }
          frame True {
            # "Turn it off...."
            # "FIELD POSITION\nGRAPH"
            # "Inches/Sec"
            # "Inches"
            # "in meters"
            # "trajectory \nmeters, radians"
            n348 = local read "outTRAJECTORY_CONFIG"() -> (w440:T2)
            n349 = local read "Track Width M"() -> (w438:dbl)
            n350 = local read "Use Diff Drive\nKinematic\nConstraint"() -> (w436:bool)
            n351 = local read "DIFF_DRIVE_KINEMATICS"() -> (w437:T1)
            n352 = local read "MaxVelocity M/S"() -> (w439:dbl)
            n353 = local read "WayPoints_M"() -> (w454:T3[])
            n354 = local read "UseWeights"() -> (w455:bool)
            n355 = call "Create_Trajectory_Make_Trajectory.vi"("TRAJECTORY_CONFIG"=w440, "Spline Type"="Spline Type", "WayPoints"=w454, "UseWeights"=w455) -> ("error out"=→"Trajectory calculation error":errorcluster, "Is Cubic"=w456:bool, "TRAJECTORY"=w443:T4)  [unwired: 5 in]
            "TRAJECTORY" <- w443
            n356 = local write "IsCubic"(w456) -> ()
            n357 = call <vilib>:"Trajectory_GetStates.vi"("TRAJECTORY"=w443) -> ("States"=w452:T5[])  [unwired: 10 in]
            "Trajectory States" <- w452
            n358 = call "Create_Trajectory_Prepare_Graph.vi"("TRAJECTORY"=w443) -> ("Array"=→"Trajectory Data":cluster{dbl[], dbl[]}[])  [unwired: 10 in]
            n359 = call "Create_Trajectory_Build_Trajectory_Field_Plot.vi"("TrackWidth_Meters"=w438, "WayPoints"=w454, "States"=w452) -> ("Array"=→"Position":cluster{dbl[], dbl[]}[])  [unwired: 8 in]
            n360 = call "Create_Trajectory_Check_Diff_Drive_Max_Speed.vi"("Use Diff Drive\nKinematic\nConstraint"=w436, "Max Speed M/S"=w439, "DIFF_DRIVE_KINEMATICS"=w437, "States"=w452) -> ("Inches/Second"=→"differential \ndrive \nmax speed":dbl, "Max Speed Exceeded"=w453:bool)  [unwired: 6 in]
            n361 = Array Size(array=w452) -> (size(s)=w448:i32)
            "Traj States\nSize" <- w448
            n362 = Not(x=w453) -> (.not. x?=w450:bool)
            n363 = Greater Than 0?(x=w448) -> (x > 0?=w449:bool)
            n364 = And(x=w449, y=w450) -> (x .and. y?=→"Trajectory\nCompleted\nError Free":bool)
            n365 = local write "Calculate\nTrajectory"(FALSE ("Calculate\nTrajectory")) -> ()
          }
        }
      }
      event "Position": Cursor Grab {
        # "Remember which one is selected"
        # "Grab a waypoint"
        n366 = event-data() -> ("CursIdx"=w457:i32)  [unwired: 1 in, 8 out]
        n367 = local write "Index"(w457) -> ()
      }
      event "Position": Cursor Release {
        # "If there are 2 or more waypoints, recalc the trajectory..."
        # "Don't forget the last selected cursor.."
        n368 = event-data() -> ()  [unwired: 1 in, 9 out]
        n369 = disable-structure shown="Disabled" {
          frame Disabled {
            n370 = local write "Index"(-1 ("Index")) -> ()
          }
          frame Enabled {
          }
        }
        n371 = local read "Units Selector"() -> (w459:T10)
        n372 = local read "WayPoints"() -> (w460:T3[])
        n373 = call "Create_Trajectory_All_WP_Units_To_Meters.vi"("Units Selector"=w459, "WayPoints"=w460) -> ("Array"=w458:T3[])  [unwired: 9 in]
        n374 = Array Size(array=w458) -> (size(s)=w461:i32)
        n375 = local write "WayPoints_M"(w458) -> ()
        n376 = Greater Or Equal?(x=w461, y=2) -> (x >= y?=w462:bool)
        n377 = case shown="True" w462 {
          frame False {
          }
          frame True {
            n378 = property on="Calculate\nTrajectory" class="Bool (strict)"("Val(Sgnl)"=TRUE ("Value (Signaling)")) -> ()  [unwired: 2 in, 2 out]
          }
        }
      }
      event "Position": Cursor Move {
        # "#NOTE Probably can use CursIdx here.   We keep our own index so that we can still change the last selected item even if it isn't selected any more."
        n379 = event-data() -> ("CursLoc"=w466:cluster{"X":dbl, "Y":dbl})  [unwired: 1 in, 8 out]
        n380 = local read "Index"() -> (w468:i32)
        n381 = Greater Or Equal To 0?(x=w468) -> (x >= 0?=w467:bool)
        n382 = case shown="True" w467 {
          tunnel: w468 -> [w479 _]
          tunnel: w466 -> [w477 _]
          frame True {
            n383 = Unbundle By Name(w477) -> ("X"=w476:dbl, "Y"=w475:dbl)
            n384 = local read "WayPoints"() -> (w478:T3[])
            n385 = local read "Units Selector"() -> (w470:T10)
            n386 = in-place {
              in-place-border: w476 -> [w484]
              in-place-border: w475 -> [w483]
              in-place-border: w470 -> [w481]
              n387 = in-place-array #4(w478, w479) -> (w485:T3)
              n388 = in-place {
                in-place-border: w484 -> [w490]
                in-place-border: w483 -> [w489]
                in-place-border: w481 -> [w486]
                n389 = in-place-cluster #5(w485) -> ()  [unwired: 2 out]
                n390 = call "Create_Trajectory_Value_Inches_To_Units.vi"("Units Selector"=w486, "Inches"=w490) -> ("Units"=w487:dbl)  [unwired: 9 in]
                n391 = call "Create_Trajectory_Value_Inches_To_Units.vi"("Units Selector"=w486, "Inches"=w489) -> ("Units"=w488:dbl)  [unwired: 9 in]
                n392 = in-place-cluster #5("X"=w487, "Y"=w488) -> (w482:T3)
              }
              n393 = in-place-array #4(w482) -> (w471:T3[])  [unwired: 1 out]
            }
            n394 = call "Create_Trajectory_All_WP_Units_To_Meters.vi"("Units Selector"=w470, "WayPoints"=w471) -> ("Array"=w469:T3[])  [unwired: 9 in]
            n395 = local write "WayPoints"(w471) -> ()
            n396 = Array Size(array=w469) -> (size(s)=w474:i32)
            n397 = local write "WayPoints_M"(w469) -> ()
            n398 = Greater Or Equal?(x=w474, y=2) -> (x >= y?=w472:bool)
            n399 = case shown="True" w472 {
              frame False {
              }
              frame True {
                n400 = property on="Calculate\nTrajectory" class="Bool (strict)"("Val(Sgnl)"=TRUE ("Value (Signaling)")) -> ()  [unwired: 2 in, 2 out]
              }
            }
          }
          frame False {
          }
        }
      }
      event "Position": Mouse Wheel {
        # "#NOTE Added modifier to allow changing the \nweight if the CTRL key is pressed while moving\nthe mouse wheel."
        # "This gives +/- 1"
        # "Update the waypoint heading....\n\nIf the CTRL key is also pressed\nthen update the weight value \ninstead."
        n401 = event-data() -> ("Delta"=w493:i32, "PlatMods"=w492:T32)  [unwired: 1 in, 8 out]
        n402 = Unbundle By Name(w492) -> ("Ctrl"=w491:bool)
        n403 = local read "Index"() -> (w496:i32)
        n404 = Greater Or Equal To 0?(x=w496) -> (x >= 0?=w495:bool)
        n405 = To Double Precision Float(number=w493) -> (double precision float=w494:dbl)
        n406 = case shown="True" w495 {
          tunnel: w496 -> [w506 _]
          tunnel: w494 -> [w504 _]
          tunnel: w491 -> [w497 _]
          frame True {
            n407 = local read "WayPoints"() -> (w505:T3[])
            n408 = case shown="False" w497 {
              tunnel: w506 -> [w509 w525]
              tunnel: w505 -> [w510 w524]
              tunnel: w504 -> [w508 w523]
              tunnel: [w507 w522] -> w501
              frame True {
                n409 = in-place {
                  in-place-border: w508 -> [w511]
                  n410 = in-place-array #6(w510, w509) -> (w513:T3)
                  n411 = in-place {
                    in-place-border: w511 -> [w516]
                    w520 = 0.01  # Low Limit
                    # "Weight can't be zero."
                    # "Adjust weight"
                    n412 = in-place-cluster #7(w513) -> ("WEIGHT"=w521:dbl)
                    n413 = Multiply(x=0.1, y=w516) -> (x*y=w515:dbl)
                    n414 = Add(x=w521, y=w515) -> (x+y=w518:dbl)
                    n415 = call <vilib>:"MathUtil_Clamp.vi"("High Limit"=inf, "Low Limit"=w520, "Value"=w518) -> ("Result"=w517:dbl)  [unwired: 8 in]
                    n416 = in-place-cluster #7("WEIGHT"=w517) -> (w512:T3)
                  }
                  n417 = in-place-array #6(w512) -> (w507:T3[])  [unwired: 1 out]
                }
              }
              frame False {
                n418 = in-place {
                  in-place-border: w523 -> [w526]
                  n419 = in-place-array #8(w524, w525) -> (w528:T3)
                  n420 = in-place {
                    in-place-border: w526 -> [w533]
                    # "Make it a heading"
                    n421 = in-place-cluster #9(w528) -> ("ANGLE"=w534:dbl)
                    n422 = Add(x=w534, y=w533) -> (x+y=w532:dbl)
                    n423 = call <vilib>:"MathUtil_InputModulus.vi"("Maximum_Input"=180.0, "Minimum_Input"=-180.0, "Input"=w532) -> ("modulus"=w529:dbl)  [unwired: 8 in]
                    n424 = in-place-cluster #9("ANGLE"=w529) -> (w527:T3)
                  }
                  n425 = in-place-array #8(w527) -> (w522:T3[])  [unwired: 1 out]
                }
              }
            }
            n426 = local read "Units Selector"() -> (w498:T10)
            n427 = local write "WayPoints"(w501) -> ()
            n428 = call "Create_Trajectory_All_WP_Units_To_Meters.vi"("Units Selector"=w498, "WayPoints"=w501) -> ("Array"=w499:T3[])  [unwired: 9 in]
            n429 = Array Size(array=w499) -> (size(s)=w500:i32)
            n430 = local write "WayPoints_M"(w499) -> ()
            n431 = Greater Or Equal?(x=w500, y=2) -> (x >= y?=w502:bool)
            n432 = case shown="True" w502 {
              frame False {
              }
              frame True {
                n433 = property on="Calculate\nTrajectory" class="Bool (strict)"("Val(Sgnl)"=TRUE ("Value (Signaling)")) -> ()  [unwired: 2 in, 2 out]
              }
            }
          }
          frame False {
          }
        }
      }
      event "Add New\nWaypoint": Value Change {
        # "If  Index < 0 or index == size-1\n     put at end\nelse"
        # "#TODO   If this is the first then put in the middle of screen.....\n                                    DONE\n                 If not at end then put in the middle of prev and next\n                                    DONE\n                 If new at end  -- if room -- then put X+24, Y, \n                                else put X, Y+/- 24 towards middle.\n                                    NOT DONE - may not really need."
        n434 = event-data() -> ("NewVal"=w536:bool)  [unwired: 1 in, 5 out]
        n435 = case shown="True" w536 {
          frame False {
          }
          frame True {
            # "Add a waypoint after the current one.."
            # "If something selected\nthen add after the\nselected item.  If nothing\nselected add to the end."
            n436 = local read "WayPoints"() -> (w546:T3[])
            n437 = local read "Index"() -> (w545:i32)
            n438 = Greater Or Equal To 0?(x=w545) -> (x >= 0?=w565:bool)
            n439 = Array Size(array=w546) -> (size(s)=w556:i32)
            n440 = local read "Units Selector"() -> (w544:T10)
            n441 = Increment(x=w545) -> (x+1=w563:i32)
            n442 = Decrement(x=w556) -> (x-1=w555:i32)
            n443 = Select(t=w563, s=w565, f=w556) -> (s? t:f=w564:i32)
            n444 = Less?(x=w545, y=w555) -> (x < y?=w553:bool)
            n445 = Greater Or Equal To 0?(x=w545) -> (x >= 0?=w554:bool)
            n446 = Greater Or Equal?(x=w556, y=2) -> (x >= y?=w552:bool)
            n447 = local read "Reverse"() -> (w537:bool)
            n448 = Compound Arithmetic op=AND(w554, w553, w552) -> (w551:bool)
            n449 = case shown="True" w551 {
              tunnel: [315.0 ("X") w589] -> w548
              tunnel: [162.0 ("Y") w588] -> w547
              tunnel: w546 -> [_ w599]
              tunnel: w545 -> [_ w597]
              tunnel: w544 -> [_ w583]
              tunnel: [0.0 ("Y") w585] -> w538
              tunnel: w537 -> [_ w572]
              frame False {
                # "Y inches"
                # "x inches"
                # "Angle  Deg"
                # "Put the cursor\nin the middle of the\nfield."
              }
              frame True {
                w592 = 0.5 ("x")
                # "Ang deg"
                # "Y inch"
                # "X inch"
                # "Put it in the middle of our two\npoints..."
                n450 = Increment(x=w597) -> (x+1=w598:i32)
                n451 = Index Array(array=w599, index #1=w597, index #2=w598) -> (element #1=w596:T3, element #2=w595:T3)
                n452 = Unbundle By Name(w596) -> ("X"=w579:dbl, "Y"=w581:dbl)
                n453 = Unbundle By Name(w595) -> ("X"=w580:dbl, "Y"=w582:dbl)
                n454 = Add(x=w581, y=w582) -> (x+y=w594:dbl)
                n455 = Subtract(x=w582, y=w581) -> (x-y=w578:dbl)
                n456 = Subtract(x=w580, y=w579) -> (x-y=w577:dbl)
                n457 = Add(x=w579, y=w580) -> (x+y=w593:dbl)
                n458 = Inverse Tangent (2 Input)(1:w577, 2:w578) -> (0:w574:dbl)
                n459 = Multiply(x=w592, y=w594) -> (x*y=w591:dbl)
                n460 = Multiply(x=w592, y=w593) -> (x*y=w590:dbl)
                n461 = Add(x=3.141592653589793, y=w574) -> (x+y=w573:dbl)
                n462 = Select(t=w573, s=w572, f=w574) -> (s? t:f=w576:dbl)
                n463 = call "Create_Trajectory_Value_Units_To_Inches.vi"("Units Selector"=w583, "Units"=w590) -> ("Inches"=w589:dbl)  [unwired: 9 in]
                n464 = call "Create_Trajectory_Value_Units_To_Inches.vi"("Units Selector"=w583, "Units"=w591) -> ("Inches"=w588:dbl)  [unwired: 9 in]
                n465 = call <vilib>:"Conv_Radians_Deg.vi"("Radians"=w576) -> ("Degrees"=w584:dbl)  [unwired: 10 in]
                n466 = call <vilib>:"MathUtil_InputModulus.vi"("Maximum_Input"=180.0, "Minimum_Input"=-180.0, "Input"=w584) -> ("modulus"=w585:dbl)  [unwired: 8 in]
              }
            }
            n467 = call "Create_Trajectory_Value_Inches_To_Units.vi"("Units Selector"=w544, "Inches"=w548) -> ("Units"=w559:dbl)  [unwired: 9 in]
            n468 = call "Create_Trajectory_Value_Inches_To_Units.vi"("Units Selector"=w544, "Inches"=w547) -> ("Units"=w558:dbl)  [unwired: 9 in]
            n469 = Bundle By Name(cluster=T15 {"Name"="Cursor", "Color"=915580, "Style"=4, "Point Style"=2, "Name Visible"=FALSE, "Allow Drag"=TRUE, "Cursor Mode"=0, "Plot"=0, "Index"=0, "Position"={"X"=315.0, "Y"=162.0}, "X Scale"=0, "Y Scale"=0, "Watch Plots"=[], "Watch All Plots"=FALSE, "Plot Area"=0, "Label Offset"={"X"=0.0, "Y"=0.0}} ("new element/subarray"), "Position.X"=w548, "Position.Y"=w547) -> (w549:T15)
            n470 = property on="Position" class="XYGraph (strict)"() -> ("CrsrList"=w566:T13)  [unwired: 2 in, 2 out]
            n471 = Bundle By Name(cluster=T3 {"X"=315.0, "Y"=162.0, "ANGLE"=0.0, "WEIGHT"=0.0} ("new element/subarray"), "X"=w559, "Y"=w558, "ANGLE"=w538, "WEIGHT"=0.2) -> (w560:T3)
            n472 = Insert Into Array(array=w546, index=w564, new element=w560) -> (w562:T3[])
            n473 = Insert Into Array(array=w566, index=w564, new element=w549) -> (w567:T13)
            n474 = call "Create_Trajectory_All_WP_Units_To_Meters.vi"("Units Selector"=w544, "WayPoints"=w562) -> ("Array"=w543:T3[])  [unwired: 9 in]
            n475 = local write "Index"(w564) -> ()
            n476 = local write "WayPoints"(w562) -> ()
            n477 = local write "WayPoints_M"(w543) -> ()
            n478 = property on="Position" class="XYGraph (strict)"("CrsrList"=w567) -> ()  [unwired: 2 in, 2 out]
            n479 = Array Size(array=w543) -> (size(s)=w542:i32)
            n480 = Greater Or Equal?(x=w542, y=2) -> (x >= y?=w540:bool)
            n481 = case shown="True" w540 {
              frame False {
              }
              frame True {
                n482 = property on="Calculate\nTrajectory" class="Bool (strict)"("Val(Sgnl)"=TRUE ("Value (Signaling)")) -> ()  [unwired: 2 in, 2 out]
              }
            }
          }
        }
      }
      event "WayPoints": Value Change {
        # "Something was typed into a waypoint value.   I think this means that\na row could have been added or deleted too.....\n\nIn this case just:\n\n -- get all the values\n  -- build the Waypoints_M data\n  -- build all the cursors\n  -- trigger the trajectory be rebuilt (if 2 or more waypoints.)"
        n483 = event-data() -> ()  [unwired: 1 in, 6 out]
        n484 = flat-sequence {
          frame #0 {
            n485 = local read "Units Selector"() -> (w605:T10)
            n486 = call "Create_Trajectory_All_WP_Units_To_Meters.vi"("Units Selector"=w605, "WayPoints"="WayPoints") -> ("Array"=w602:T3[])  [unwired: 9 in]
            n487 = call "Create_Trajectory_All_WP_Meters_To_Units.vi"("Units Selector"=TrajCreateUnitsENUM."Inches", "WayPoints_M"=w602) -> ("outWayPoints_UNITS"=w601:T3[])  [unwired: 9 in]
            n488 = for {
              tunnel: w601 -> [w609] mode=indexing
              tunnel: [w606] -> w604 mode=indexing
              n489 = Unbundle By Name(w609) -> ("X"=w608:dbl, "Y"=w607:dbl)
              n490 = Bundle By Name(cluster=T15 {"Name"="Cursor", "Color"=915580, "Style"=4, "Point Style"=2, "Name Visible"=FALSE, "Allow Drag"=TRUE, "Cursor Mode"=0, "Plot"=0, "Index"=0, "Position"={"X"=315.0, "Y"=162.0}, "X Scale"=0, "Y Scale"=0, "Watch Plots"=[], "Watch All Plots"=FALSE, "Plot Area"=0, "Label Offset"={"X"=0.0, "Y"=0.0}} ("new element/subarray"), "Position.X"=w608, "Position.Y"=w607) -> (w606:T15)
            }
            n491 = local write "WayPoints_M"(w602) -> ()
            n492 = property on="Position" class="XYGraph (strict)"("CrsrList"=w604) -> ()  [unwired: 2 in, 2 out]
          }
          frame #1 {
            n493 = property on="Calculate\nTrajectory" class="Bool (strict)"("Val(Sgnl)"=TRUE ("Value (Signaling)")) -> ()  [unwired: 2 in, 2 out]
          }
        }
      }
      event "Remove Current\nWaypoint": Value Change {
        n494 = event-data() -> ("NewVal"=w612:bool)  [unwired: 1 in, 5 out]
        n495 = case shown="True" w612 {
          frame False {
          }
          frame True {
            # "Only do anyting\nif there is something\nto remove."
            n496 = local read "Index"() -> (w614:i32)
            n497 = Greater Or Equal To 0?(x=w614) -> (x >= 0?=w613:bool)
            n498 = case shown="True" w613 {
              tunnel: w614 -> [_ w615]
              frame False {
              }
              frame True {
                # "Remove cursoe"
                n499 = flat-sequence {
                  tunnel: w615 -> [w625]
                  frame #0 {
                    # "Just in case"
                    # "Remove Waypoint"
                    n500 = local read "WayPoints"() -> (w624:T3[])
                    n501 = property on="Position" class="XYGraph (strict)"() -> ("CrsrList"=w623:T13)  [unwired: 2 in, 2 out]
                    n502 = local read "Units Selector"() -> (w616:T10)
                    n503 = Delete From Array(array=w624, length=1, index=w625) -> (array with subset deleted=w619:T3[])  [unwired: 1 out]
                    n504 = Delete From Array(array=w623, length=1, index=w625) -> (array with subset deleted=w622:T13)  [unwired: 1 out]
                    n505 = local write "WayPoints"(w619) -> ()
                    n506 = call "Create_Trajectory_All_WP_Units_To_Meters.vi"("Units Selector"=w616, "WayPoints"=w619) -> ("Array"=w617:T3[])  [unwired: 9 in]
                    n507 = property on="Position" class="XYGraph (strict)"("CrsrList"=w622) -> ()  [unwired: 2 in, 2 out]
                    n508 = Decrement(x=w625) -> (x-1=w620:i32)
                    n509 = Array Size(array=w617) -> (size(s)=w618:i32)
                    n510 = local write "WayPoints_M"(w617) -> ()
                    n511 = local write "Index"(w620) -> ()
                    n512 = Greater Or Equal?(x=w618, y=2) -> ()  [unwired: 1 out]
                  }
                  frame #1 {
                    # "#NOTE Try and recalc trajectory\neven if there are too few waypoints."
                    n513 = property on="Calculate\nTrajectory" class="Bool (strict)"("Val(Sgnl)"=TRUE ("Value (Signaling)")) -> ()  [unwired: 2 in, 2 out]
                  }
                }
              }
            }
          }
        }
      }
    }
    n514 = case shown="True" "Terminate" {
      frame False {
      }
      frame True {
        # "The end program button was pressed."
        n515 = disable-structure shown="Default" {
          frame condition #0 (active) {
            n516 = Stop(stop? (T)=TRUE) -> ()
          }
          frame condition #1 {
            n517 = Quit LabVIEW(quit? (T)=TRUE) -> ()
          }
        }
      }
    }
  }
